vi "AlliGator Files Actions.vi"(0 "AlliGator Q Elements in":T5[](array[typedef]), 1 "VI in":refnum<vi>, 2 "Script in":bool, 5 "AlliGator IV DVR":refnum<data-value>, 7 "AlliGator Q Event in":T6=enum."GUI:Idle", 9 "Data":variant, 11 "error in (no error)":errorcluster, 12 "AlliGator Ctrl Refnums":T7) -> (3 "Script out":bool, 4 "AlliGator Q Elements out":T5[](array[typedef]), 6 "AlliGator IV DVR":refnum<data-value>, 10 "[Notebook Message]":T2[](array[typedef]) {"Message Style"."Text Alignment" items=["Left", "Right", "Center"]}, 15 "error out":errorcluster)   [LabVIEW 2021, in "AlliGator Action Engine.lvlib"]
doc: "Processes AlliGator files-related actions."
uses:
  AlliGator Action Engine.lvlib
  AlliGator Q Event.ctl
  AlliGator Ctrl Refnums.ctl
  AlliGator Other Ctrl Refnums.ctl
  AlliGator State Indicator.ctl
  AlliGator Phasor Plot Ctrl Refnums.ctl
  AlliGator Phasor Graph Ctrl Refnums.ctl
  Phasor/Phasor Calibration Type.ctl
  AlliGator Dataset Ctrl Refnums.ctl
  AlliGator Displayed Image.ctl
  AlliGator Registered Events Ctrl Refnums.ctl
  AlliGator Image Histogram Control Refnums.ctl
  Histograms/Linear Histogram Options.ctl
  Histograms/Histogram Bin Option.ctl
  Histograms/Histogram Bin Position.ctl
  AlliGator Decay Fit Map Control Refnums.ctl
  Fits/IRF(X)PSED/Decay Fit Parameters & Derived Quantities List.ctl
  AlliGator Q Element.ctl
  AlliGator Internal Variables v2.ctl
  <vilib>/vision/Image Controls.llb/IMAQ Image.ctl
  AlliGator Gate Image Set.ctl
  AlliGator FLI Dataset Type.ctl
  AlliGator Data Series Type.ctl
  AlliGator Dataset Channel.ctl
  AlliGator Gate Arithmetic.ctl
  Image/Named ROI Description.ctl
  AlliGator Decay Metadata v3.ctl
  AlliGator Decay Background Subtraction Info.ctl
  AlliGator Baseline Subtraction Method.ctl
  Graphs/XY Graph/XY Graph Plot Shift Parameters.ctl
  Graphs/XY Graph/XY Graph Plot Shift Method.ctl
  AlliGator Decay Extrapolation Parameters.ctl
  Phasor/Calibration Phasor (m, phi).ctl
  Phasor/Phasor Reference Series.ctl
  Phasor/Phasor Calibration Map v2.ctl
  Phasor/Phasor (g, s).ctl
  AlliGator Raw Phasor Plot Data v4.ctl
  Phasor/Phasor Standard Deviation Options.ctl
  AlliGator Phasor Multi-Harmonic Data.ctl
  Phasor/Phasor Harmonic Data.ctl
  AlliGator Decay Fit Options & Parameters v2.ctl
  Fits/IRF(X)PSED/Decay Fit Options v2.ctl
  Fits/Decay Convolution/Decay Model.ctl
  Fits/Residual Type.ctl
  Fits/IRF(X)PSED/Fit Weights Type.ctl
  Fits/Non-linear Fitting Method v2.ctl
  Fits/Fit Calculation Method.ctl
  Fits/Non-linear Fitting Algorithm.ctl
  AlliGator Decay Fit Parameter Constraints 2.ctl
  Fits/IRF(X)PSED/Decay Fit Parameters In List.ctl
  Fits/IRF(X)PSED/MLE Baseline Offset Type.ctl
  AlliGator Decay Preprocessing Parameters.ctl
  Notebook/Notebook Message Object.ctl
  Rich Text Box/Text Formatting.ctl
  Rich Text Box/Text Colors.ctl
  AlliGator Windows List.ctl
  Alligator Elements Order in Action Stack.ctl
  AlliGator Export Dataset Options.ctl
  AlliGator Variables List.ctl
  AlliGator Load Dataset Options.ctl
  AlliGator Single Image File Info.ctl
  AlliGator Image Type.ctl
  AlliGator Folder Selection.ctl
  AlliGator Select Folder Mode.ctl
  AlliGator Data Load & Process Options.ctl
  AlliGator Data Information.ctl
  AlliGator Gates to Skip.ctl
  AlliGator Define Gates to.ctl
  AlliGator Gates to Keep.ctl
  AlliGator Source Image Settings.ctl
  AlliGator Low Count Pixels Rejection Options.ctl
  AlliGator High Count Pixels Rejection Options.ctl
  AlliGator Image Smoothing Options.ctl
  Arrays/Kernel Type.ctl
  Arrays/Smoothing Algorithm.ctl
  AlliGator Image Binning Options.ctl
  AlliGator Decay Preprocessing Options.ctl
  AlliGator Background Subtraction Parameters.ctl
  AlliGator Settings List.ctl
  AlliGator Globals.vi
  AlliGator Add Action Array to Stack.vi
  Variant/Variant to Data/Variant to I32.vi
  Variant/Variant to Data/Variant to Path.vi
  AlliGator Add Single Action to Stack.vi
  Variant/Variant to Data/Variant to DBL.vi
  Variant/Variant to Data/Variant to Data.lvlib
  AlliGator GUI.lvlib
  Utilities/Utilities.lvlib
  GUI/GUI.lvlib
  AlliGator Files.lvlib
  AlliGator Source Image.lvlib
  AlliGator Scripts.lvlib
  Graphs/XY Graph/XY Graph Add-Ons.lvlib
  AlliGator Decay Preprocessing.lvlib
  Arrays/Arrays.lvlib
  AlliGator Settings.lvlib
  AlliGator Decay Analysis.lvlib
  AlliGator Globals, Variables & Constants.lvlib
  Rich Text Box/Rich Text Box.lvlib
  Image/Image.lvlib
  Phasor/Phasor.lvlib
  AlliGator Decay Fit Parameter Map.lvlib
  AlliGator Phasor Graph.lvlib
  AlliGator Phasor Plot.lvlib
  Fits/Fits.lvlib
  AlliGator Decay Fit.lvlib
  AlliGator Internal Variables.lvlib
  AlliGator Dual-Channel Datasets.lvlib
  Histograms/Histogram Window.lvlib
  Notebook/Notebook.lvlib
panel:
  in  "Displayed Image 2":T1=enum."Sum of All Gates" caption="Displayed Image"
  in  "Displayed Image":T1=enum."Sum of All Gates"
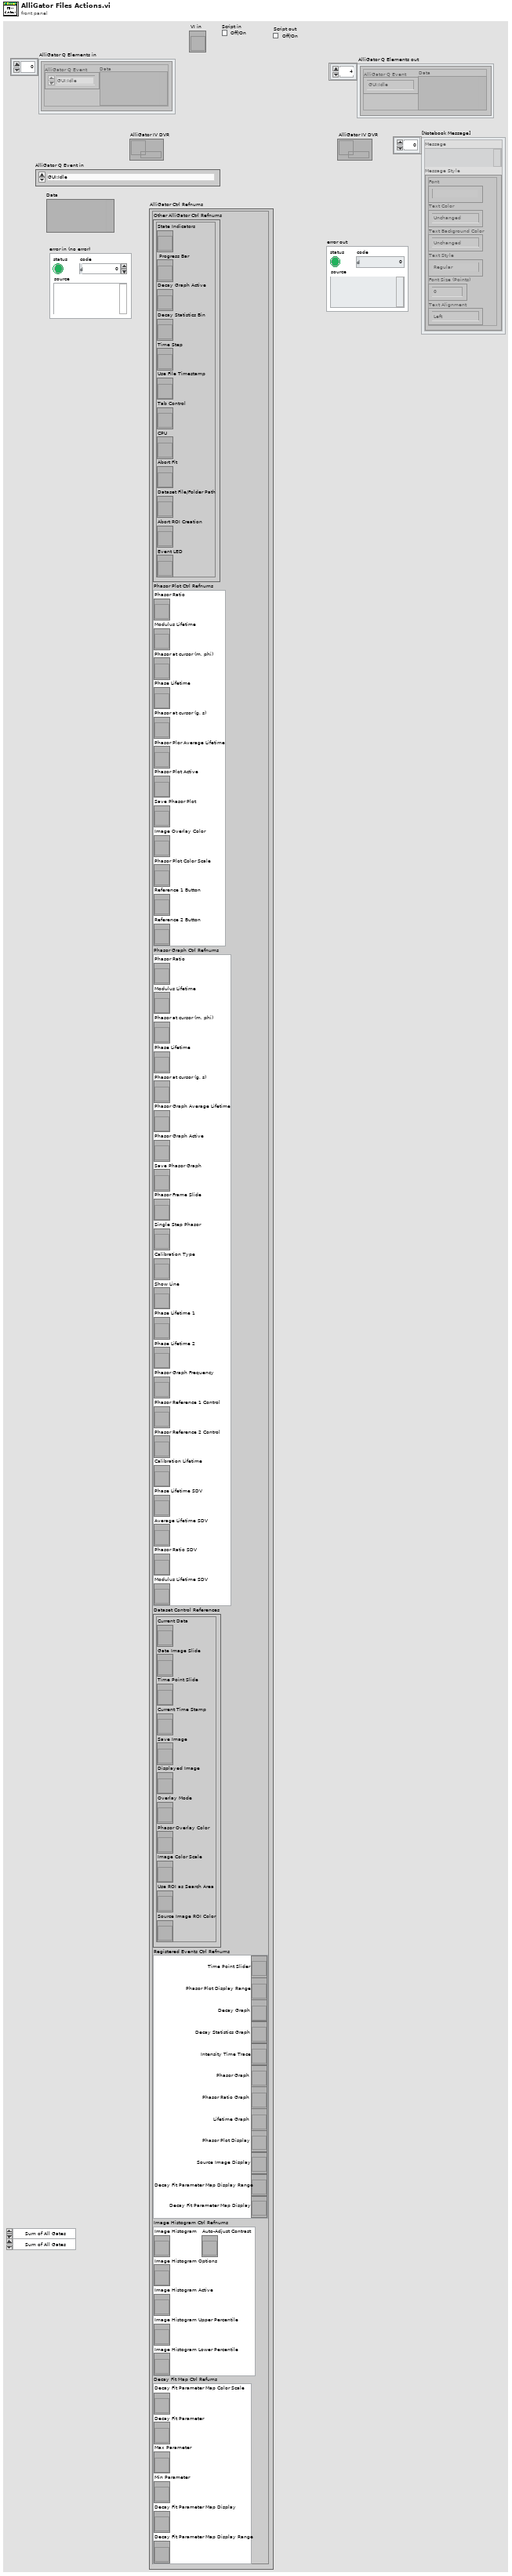
[diagram p1: front panel]
types:
  T1 = typedef "AlliGator Source Image.lvlib/AlliGator Displayed Image.ctl" = enum16{"Single Gate", "Sum of All Gates", "Max of All Gates", "Min of All Gates", "-", "White Ligth Image", "Mask Image"}
  T2 = typedef "Notebook.lvlib/Notebook Message Object.ctl" = cluster{"Message":string, "Message Style":T3}
  T3 = typedef "Rich Text Box.lvlib/Text Formatting.ctl" = cluster{"Font":string, "Text Color":T4, "Text Background Color":T4, "Text Style":enum16{"Regular", "Bold", "Italic", "Underline", "Strikeout"}, "Font Size (Points)":dbl, "Text Alignment":i32}
  T4 = typedef "Rich Text Box.lvlib/Text Colors.ctl" = enum16{"Unchanged", "Black", "Blue", "Brown", "Gray", "Green", "Orange", "Pink", "Red", "White"}
  T5 = typedef "AlliGator Action Engine.lvlib/AlliGator Q Element.ctl" = cluster{"AlliGator Q Event":T6, "Data":variant}
  T6 = typedef "AlliGator Action Engine.lvlib/AlliGator Q Event.ctl" = enum16{"---- Files ----", "Files:Set Batch Export Files To Save", "Files:Set Dataset Loading & Pre-processing Options", "Files:Check #Frames in Dataset", "Files:Increment Frame Index", "Files:Open Mask Image", "Files:Open White Light Image", "Files:Open Single Dataset", "Files:New Folder of Folders Selected", "Files:Load File (all Types)_Scriptable", "Files:Move Flattened Series to Folders Series", "Files:Select Folder", "Files:Load FLI Dataset", "Files:Load Swiss SPAD 1 Dataset", "Files:Load Swiss SPAD 2 Dataset", "Files:Load .sdt FLI Dataset", "Files:Load .ptu FLI Dataset", "Files:Load .bin FLI Dataset", "Files:Load Single Gate Image Folder", "Files:Load I/m/phi Dataset (deprecated)", "Files:Load Single Image", "Files:Subtract Background File", "Files:Export FLI Dataset", "Files:Load HDF5 FLI Dataset", "Files:Set Destination File Path", "Files:Save Mask Image", "Files:Batch Conversion", "Files:New Folder Selected", "Files:Close FLI Dataset", "Files:Close FLI Dataset Series", "Files:Close White Light Image", "Files:Close Mask Image", "---- FLI Dataset ----", "FLI Dataset:Channel Arithmetic", "FLI Dataset:Export Average Lifetime Map as ASCII", "FLI Dataset:Export User-Defined Quantity Map as ASCII", "FLI Dataset:Python Function FLI Dataset Event", "FLI Dataset:ROI Analysis", "FLI Dataset:Tilted Logistic Square Gated IRF Characteristics Map", "FLI Dataset:Logistic Square Gated IRF Characteristics Map", "FLI Dataset:Square Gated IRF Characteristics Map", "FLI Dataset:Multi-ROI Single-Pixel Phasor Analysis", "FLI Dataset:Multi-ROI Single-Pixel NLSF Analysis", "FLI Dataset:All ROIs IRF Extraction", "FLI Dataset:All ROIs Decay Fit Non-Interactive (Fast + Individual IRF)", "FLI Dataset:All ROIs Phasor Analysis", "FLI Dataset:All ROIs Decay Fit", "FLI Dataset:Fluorescence Decay Statistics", "FLI Dataset:Update Decay Statistics Graph", "FLI Dataset:Get Decay from ROI", "FLI Dataset:All ROIs Average Lifetimes", "---- FLI Dataset Series ----", "FLI Dataset Series:Sum All Datasets in Series", "FLI Dataset Series:Add Dataset to Accumulated Dataset", "FLI Dataset Series:Display Accumulated Dataset", "FLI Dataset Series:Clear Dataset Series Sum", "FLI Dataset Series:Time-Series Analysis (NLSF)", "FLI Dataset Series:Time-Series Analysis (Phasor)", "---- Image ----", "Image:Update Image Profile Plots", "Image:Image Histogram Cursor Move", "Image:Image Histogram", "Image:Image Contrast", "Image:Set Image Histogram Cursor Move Flag", "Image:Clear Image Overlay", "Image:Use ROI as Search Area", "Image:Set ROI Diameter", "Image:Save Image Data as TIFF", "Image:Save Displayed Image with Overlay", "Image:Save Image Overlay Only", "Image:Save Image as Hot Pixel Mask", "Image:Change Source Image Color Palette", "Image:Copy Image to Clipboard", "Image:Source Image ROI Selection", "Image:Delete All ROIs", "Image:Delete All Unselected ROIs", "Image:Delete ROI", "Image:Merge All ROIs", "Image:Store ROI", "Image:Source Image ROI Storage", "Image:Export ROI Description to Notebook", "Image:Save ROI", "Image:Load ROI", "Image:Paste ROI Definition", "Image:Clear ROI", "Image:Identify ROIs in Mask Image", "Image:Create Complementary ROI", "Image:Create Contour ROI", "Image:Create ROI(s) from Pixels with Peak above Min_Scriptable", "Image:Create ROI(s) from Pixels with Intensity above Min_Scriptable", "Image:Compute ROI Statistics", "Image:Delete ROI(s) based on ROI Characteristics", "Image:Create ROI Grid", "Image:ROI to Individual Pixel ROIs", "Image:Python Function Source Image Event", "Image:Show Phasor Calibration Map ROI Centers", "Image:Convert ROI to Mask Image", "Image:Mouse Move", "Image:Mouse Up", "Image:Set Source Image Mouse Move Flag", "Image:Add Scale Bar Overlay", "Image:Delete Existing ROIs Option", "---- Decay ----", "Decay:Clear IRF/Reference Plot", "Decay:Clear Local IRFs", "Decay:Add Decay to Graph", "Decay:Smoothen Plot", "Decay:Smoothen Plot Tail", "Decay:Average Selected Plots", "Decay:Extract IRF", "Decay:Optimal IRF Extraction", "Decay:Threshold IRF", "Decay:Fit to Model IRF", "Decay:Fit IRF to Square Gate", "Decay:Fit IRF to Logistic Square Gate", "Decay:Fit IRF to Tilted Logistic Square Gate", "Decay:Create Bounding Cursors Set", "Decay:Export Bounding Cursors Definition to Notebook", "Decay:Denoise Plot", "Decay:Compute Cumulative Function", "Decay:Use as Reference Decay", "Decay:Show Reference Decay/IRF", "Decay:Extrapolate Decay", "Decay:Create Head & Tail Bounding Cursors", "Decay:Store Cursor-defined Head & Tail Fractions", "Decay:Rebin Plot", "Decay:1-Normalize Decay", "Decay:[0-1]-Normalize Plot", "Decay:Straighten Decay", "Decay:Shift Decay", "Decay:Fold Decay", "Decay:Fit Decay", "Decay:Global Fit of Selected Decays", "Decay:Post Global Fit Script", "Decay:Add Global Fit Parameters to Graph", "Decay:Add Decay Parameter(s) to Plot (Graph)", "Decay:Export Decay to Phasor Graph", "Decay:Plot Decay Shifts", "Decay:Compute Average Lifetime", "Decay:Plot Convolution", "Decay:Graph Tip Strip Update", "---- Decay Statistics ----", "Decay Statistics:Tip Strip Update", "---- Intensity Time Trace ----", "Intensity Time Trace:Use File Timestamp", "Intensity Time Trace:Load Intensity Corrections File", "Intensity Time Trace:Clear Intensity Corrections File", "Intensity Time Trace:Tip Strip Update", "---- Phasor Plot ----", "Phasor Plot:Build Phasor Plot", "Phasor Plot:Change Phasor Plot Color Palette", "Phasor Plot:Adjust Phasor Plot Display Range", "Phasor Plot:Highlight Image ROI in Phasor Plot", "Phasor Plot:Save Phasor Plot Image with Overlay", "Phasor Plot:Export Complex Phasor Map", "Phasor Plot:Export Phasor Ratio Map", "Phasor Plot:Export Average Lifetime Map", "Phasor Plot:Compute Phase Lifetime Histogram", "Phasor Plot:Compute Phasor Ratio Histogram", "Phasor Plot:Compute Phase Lifetime vs Intensity Scatter Plot", "Phasor Plot:Weber 2-Component Decomposition", "Phasor Plot:Update Phasor Color Map Vertices", "Phasor Plot:Clear Phasor Overlay", "Phasor Plot:Use Segment Extremities as References", "Phasor Plot:Use UC/Segment Intersections as References", "Phasor Plot:Use UC/Principal Axis Intersections as References", "Phasor Plot:Use UC/Linear Fit Intersections as References", "Phasor Plot:Update Phasor Plot Reference", "Phasor Plot:Show Local Phasor Info in Phasor Plot", "Phasor Plot:Update Phasor Plot State", "Phasor Plot:Phasor Plot ROI Storage", "Phasor Plot:Phasor Plot ROI Selection", "Phasor Plot:Python Function Phasor Plot Event", "Phasor Plot:Overlay Phasor ROI, Ratio or Map in Source Image", "Phasor Plot:Compute Decay of Selected Phasors", "Phasor Plot:Phasor at Image Pixel", "Phasor Plot:Mouse Move", "Phasor Plot:Mouse Up", "Phasor Plot:Display Range Mouse Move", "Phasor Plot:Set Mouse Move Flag", "---- Phasor Graph ----", "Phasor Graph:Calibrated Phasor Map Series", "Phasor Graph:Whole Image Phasor Scatter Plot (Todo)", "Phasor Graph:Get Phasor Value", "Phasor Graph:Create New Phasor Plot Dialog", "Phasor Graph:Update Last Phasor Value", "Phasor Graph:Update Phasor (m, phi)", "Phasor Graph:Remove Single Phasor from Plot", "Phasor Graph:Add Single Phasor to Plot", "Phasor Graph:Remove Phasor Plot", "Phasor Graph:Remove Selected Phasor Plots", "Phasor Graph:Clear Phasor Data", "Phasor Graph:Clear Phasor Graph", "Phasor Graph:Cursor Move", "Phasor Graph:Draw Cursor Connecting Line", "Phasor Graph:Clear Cursor Connecting Line", "Phasor Graph:Find UC Intersection", "Phasor Graph:Use UC/Cursor-Defined Line Intersections", "Phasor Graph:Use Selected Plots Fitted Line/UC Intersections", "Phasor Graph:Use Selected Plots Principal Axis/UC Intersections", "Phasor Graph:Show Single Phasor", "Phasor Graph:Save Single Phasor Plot", "Phasor Graph:Save All Phasor Plots", "Phasor Graph:Load Phasor Plot(s)", "Phasor Graph:Phasor Multiplication", "Phasor Graph:Compute Average Phasor", "Phasor Graph:Compute Multiple Average Phasors (Selected Plots)", "Phasor Graph:Export Single Phasor Plot Phase Lifetimes", "Phasor Graph:Phase Lifetime Trajectory", "Phasor Graph:Phase Lifetime vs Intensity Scatter Plot (deprecated)", "Phasor Graph:Parameter 2 vs Parameter 1 Scatter Plot", "Phasor Graph:Use Cursor n Location", "Phasor Graph:Set Reference n to Current Phase Lifetime Value", "Phasor Graph:Set Reference n to Lifetime Value", "Phasor Graph:Set Cursor n Location", "Phasor Graph:Save Phasor Graph Image", "Phasor Graph:Update SEPL Plot", "Phasor Graph:Export Single Phasor Plot Data", "Phasor Graph:Export Selected Phasor Plots Data", "Phasor Graph:Python Function Phasor Graph Event", "Phasor Graph:Tip Strip Update", "---- Calibration ----", "Calibration:Set Calibration Type", "Calibration:Load/Save Phasor Calibration", "Calibration:Load/Save Phasor Calibration Series", "Calibration:Load/Save Phasor Calibration Map", "Calibration:Use as Calibration", "Calibration:Compute Optimal Calibration from Phasor References", "Calibration:Clear Phasor Calibration", "Calibration:Use as Calibration Series", "Calibration:Use as Calibration Map", "Calibration:Clear Calibration Series", "Calibration:Clear Calibration Map", "Calibration:Apply Phasor Calibration", "Calibration:Update Single Plot Calibration", "Calibration:Update Multiple Plots Calibration", "Calibration:Clear Single Plot Calibration", "Calibration:Clear All Plots Calibrations", "Calibration:Clear Plot(s) Calibration(s)?", "Calibration:Phasor Calibration Maps (# Gates Series)", "---- Phasor Ratio ----", "Phasor Ratio:Clear Reference n", "Phasor Ratio:Toggle Selected Plot(s)  Lock to Reference 1", "Phasor Ratio:Use as Reference n", "Phasor Ratio:Send Reference n to Notebook", "Phasor Ratio:Toggle Selected Plot(s)  Lock to Reference 2", "Phasor Ratio:Compute Phasor Ratio at Mouse Location", "Phasor Ratio:Compute Phasor Plot's Average Phasor Ratio", "Phasor Ratio:Compute Time-Series Phasor Ratios", "Phasor Ratio:Fit Line to Phasor Ratio Plot", "Phasor Ratio:Save References", "Phasor Ratio:Load References", "Phasor Ratio:Update Phasor Reference 1", "Phasor Ratio:Update Phasor Reference 2", "Phasor Ratio:Move Cursor n to Reference n", "Phasor Ratio:Use as Phasor Reference 1 Lifetime", "Phasor Ratio:Use as Phasor Reference 2 Lifetime", "Phasor Ratio:Export Phasor Ratio Map as ASCII", "Phasor Ratio:Tip Strip Update", "---- Lifetime & Other Parameters Graph ----", "Lifetime:Tip Strip Update", "---- Decay Fit Parameter Map ----", "Decay Fit Parameter Map:Export ROI NLSF Data as ASCII", "Decay Fit Parameter Map:Set Decay Fit  Parameter Map Selection", "Decay Fit Parameter Map:Build Decay Fit Parameter Map", "Decay Fit Parameter Map:Change Decay Fit Parameter Map Color Palette", "Decay Fit Parameter Map:Export Decay Fit Parameter Map Data as ASCII", "Decay Fit Parameter Map:Export All Decay Fit Parameter Maps Data as ASCII", "Decay Fit Parameter Map:Send Map Data to Lifetime Graph", "Decay Fit Parameter Map:Save Decay Fit Parameter Map Image", "Decay Fit Parameter Map:Save-Load IRFs & Fit Data", "Decay Fit Parameter Map:Update Local Decay Plots", "Decay Fit Parameter Map:Python Function Decay Fit Parameters Map Event", "Decay Fit Parameter Map:Overlay Decay Fit Parameter Map in Source Image", "Decay Fit Parameter Map:Plot Map Data vs Intensity", "Decay Fit Parameter Map:Mouse Up", "Decay Fit Parameter Map:Display Range Mouse Move", "---- Generic Graph ----", "Generic Graph:Generic XY Graph Event", "Generic Graph:Python Function XY Graph Event", "Generic Graph:New Plot", "Generic Graph:Save Plot", "Generic Graph:XY Plot Histogram", "Generic Graph:Set XY Graph Plot Name", "Generic Graph:Set Last Cursor Style", "Generic Graph:Tip Strip Update", "---- GUI ----", "GUI:Start Script", "GUI:Type of Displayed Image Changed", "GUI:Gate Image Slide Changed", "GUI:Show Busy Icon", "GUI:Show Busy Icon & Abort Button", "GUI:Hide Busy Icon", "GUI:Hide Busy Icon & Abort Button", "GUI:Abort", "GUI:End Script", "GUI:Start Timing", "GUI:End Timing", "GUI:Set State Indicator", "GUI:Send Parameters JSON Strings to Clipboard", "GUI:Set Gate Step", "GUI:Idle", "GUI:Initialization", "GUI:Quit", "GUI:Increment Dataset Index", "GUI:Set Dataset Index to -1", "GUI:Time Series Slider Moved", "GUI:Time Series Slider Changed", "GUI:Toggle Playback or Loop", "GUI:Playback Script", "GUI:Set Phasor Frequency", "GUI:Open Window", "DEBUG"}
  T7 = typedef "AlliGator GUI.lvlib/AlliGator Ctrl Refnums.ctl" = cluster{"Other AlliGator Ctrl Refnums":T8, "Phasor Plot Ctrl Refnums":T9, "Phasor Graph Ctrl Refnums":T10, "Dataset Control References":T11, "Registered Events Ctrl Refnums":T12, "Image Histogram Ctrl Refnums":T13, "Decay Fit Map Ctrl Refums":T14}
  T8 = typedef "AlliGator GUI.lvlib/AlliGator Other Ctrl Refnums.ctl" = cluster{"State Indicators":refnum<vi>, " Progress Bar":refnum<vi>, "Decay Graph Active":refnum<vi>, "Decay Statistics Bin":refnum<vi>, "Time Step":refnum<vi>, "Use File Timestamp":refnum<vi>, "Tab Control":refnum<vi>, "CPU":refnum<vi>, "Abort Fit":refnum<vi>, "Dataset File/Folder Path":refnum<vi>, "Abort ROI Creation":refnum<vi>, "Event LED":refnum<vi>}
  T9 = typedef "AlliGator GUI.lvlib/AlliGator Phasor Plot Ctrl Refnums.ctl" = cluster{"Phasor Ratio":refnum<vi>, "Modulus Lifetime":refnum<vi>, "Phasor at cursor (m, phi)":refnum<vi>, "Phase Lifetime":refnum<vi>, "Phasor at cursor (g, s)":refnum<vi>, "Phasor Plor Average Lifetime":refnum<vi>, "Phasor Plot Active":refnum<vi>, "Save Phasor Plot":refnum<vi>, "Image Overlay Color":refnum<vi>, "Phasor Plot Color Scale":refnum<vi>, "Reference 1 Button":refnum<vi>, "Reference 2 Button":refnum<vi>}
  T10 = typedef "AlliGator GUI.lvlib/AlliGator Phasor Graph Ctrl Refnums.ctl" = cluster{"Phasor Ratio":refnum<vi>, "Modulus Lifetime":refnum<vi>, "Phasor at cursor (m, phi)":refnum<vi>, "Phase Lifetime":refnum<vi>, "Phasor at cursor (g, s)":refnum<vi>, "Phasor Graph Average Lifetime":refnum<vi>, "Phasor Graph Active":refnum<vi>, "Save Phasor Graph":refnum<vi>, "Phasor Frame Slide":refnum<vi>, "Single Step Phasor":refnum<vi>, "Calibration Type":refnum<vi>, "Show Line":refnum<vi>, "Phase Lifetime 1":refnum<vi>, "Phase Lifetime 2":refnum<vi>, "Phasor Graph Frequency":refnum<vi>, "Phasor Reference 1 Control":refnum<vi>, "Phasor Reference 2 Control":refnum<vi>, "Calibration Lifetime":refnum<vi>, "Phase Lifetime SDV":refnum<vi>, "Average Lifetime SDV":refnum<vi>, "Phasor Ratio SDV":refnum<vi>, "Modulus Lifetime SDV":refnum<vi>}
  T11 = typedef "AlliGator GUI.lvlib/AlliGator Dataset Ctrl Refnums.ctl" = cluster{"Current Data":refnum<vi>, "Gate Image Slide":refnum<vi>, "Time Point Slide":refnum<vi>, "Current Time Stamp":refnum<vi>, "Save Image":refnum<vi>, "Displayed Image":refnum<vi>, "Overlay Mode":refnum<vi>, "Phasor Overlay Color":refnum<vi>, "Image Color Scale":refnum<vi>, "Use ROI as Search Area":refnum<vi>, "Source Image ROI Color":refnum<vi>}
  T12 = typedef "AlliGator GUI.lvlib/AlliGator Registered Events Ctrl Refnums.ctl" = cluster{"Time Point Slider":refnum<vi>, "Phasor Plot Display Range":refnum<vi>, "Decay Graph":refnum<vi>, "Decay Statistics Graph":refnum<vi>, "Intensity Time Trace":refnum<vi>, "Phasor Graph":refnum<vi>, "Phasor Ratio Graph":refnum<vi>, "Lifetime Graph":refnum<vi>, "Phasor Plot Display":refnum<vi>, "Source Image Display":refnum<vi>, "Decay Fit Parameter Map Display Range":refnum<vi>, "Decay Fit Parameter Map Display":refnum<vi>}
  T13 = typedef "AlliGator GUI.lvlib/AlliGator Image Histogram Control Refnums.ctl" = cluster{"Image Histogram":refnum<vi>, "Image Histogram Options":refnum<vi>, "Image Histogram Active":refnum<vi>, "Image Histogram Upper Percentile":refnum<vi>, "Image Histogram Lower Percentile":refnum<vi>, "Auto-Adjust Contrast":refnum<vi>}
  T14 = typedef "AlliGator Decay Fit Parameter Map.lvlib/AlliGator Decay Fit Map Control Refnums.ctl" = cluster{"Decay Fit Parameter Map Color Scale":refnum<vi>, "Decay Fit Parameter":refnum<vi>, "Max Parameter":refnum<vi>, "Min Parameter":refnum<vi>, "Decay Fit Parameter Map Display":refnum<vi>, "Decay Fit Parameter Map Display Range":refnum<vi>}
  T15 = typedef "AlliGator GUI.lvlib/AlliGator Windows List.ctl" = enum16{"AlliGator Window", "Settings Window", "Notebook Window", "Dataset Information Window", "Source Image ROI Manager Window", "Phasor Plot ROI Manager Window", "Phasor Harmonic Manager Window", "Histogram Window", "Image Profile Window", "Local Decay Window", "About Window", "Batch Conversion Window", "Shot Noise Influence on Average Lifetime", "Fit Method Benchmark", "AlliGator Alias Definition"}
  T16 = typedef "AlliGator Action Engine.lvlib/Alligator Elements Order in Action Stack.ctl" = enum16{"Enqueue 2 AFTER 1", "Enqueue 2 BEFORE 1"}
  T17 = typedef "AlliGator Files.lvlib/AlliGator Export Dataset Options.ctl" = cluster{"Destination File Type":string, "Dialog?":bool}
  T18 = typedef "AlliGator Files.lvlib/AlliGator Load Dataset Options.ctl" = cluster{"FLI Dataset Type":T19, "No Dialog?":bool, "File Path":path}
  T19 = typedef "AlliGator Files.lvlib/AlliGator FLI Dataset Type.ctl" = enum16{"HDF5 FLI Dataset", "Gate Image Folder", ".sdt FLI Dataset (Becker & Hickl)", ".ptu FLI Dataset (PicoQuant)", "SS1 FLI Dataset", "SS2 FLI Dataset", "I/m/phi Dataset", ".bin FLI Dataset (PicoQuant Binned)", ".bin FLI Dataset (Piccolo Binned)"}
  T20 = typedef "AlliGator Files.lvlib/AlliGator Single Image File Info.ctl" = cluster{"Image Type":T21, "Image Path":path}
  T21 = typedef "AlliGator Source Image.lvlib/AlliGator Image Type.ctl" = enum16{"White Light Image", "Mask Image"}
  T22 = typedef "AlliGator Files.lvlib/AlliGator Folder Selection.ctl" = cluster{"Folder Selection Mode":T23, "Folder Path":path}
  T23 = typedef "AlliGator Files.lvlib/AlliGator Select Folder Mode.ctl" = enum16{"Select Gate Folder", "Select Folder of Gate Folders", "Select Folder of SwissSPAD 2 Datasets", "Select Folder of .sdt FLI Datasets (Becker & Hickl)", "Select Folder of .ptu FLI Datasets (PicoQuant)", "Select Folder of .bin FLI Datasets (PicoQuant Binned)", "Select Folder of .bin FLI Datasets (Piccolo Binned)", "Select Folder of HDF5 FLI Datasets"}
  T24 = typedef "AlliGator Scripts.lvlib/AlliGator Data Load & Process Options.ctl" = cluster{"Data Information":T25, "Source Image Settings":T30, "Decay Preprocessing Options & Parameters":T37, "Clear Phasor Graph":bool}
  T25 = typedef "AlliGator Scripts.lvlib/AlliGator Data Information.ctl" = cluster{"Gates to Skip":T26, "# Gates":u32, "Gate Step":u32, "Gate Duration":dbl[unit], "Gate Separation":dbl[unit], "Pile-up Correction":bool, "Pixel Well Capacity":u32, "Define Gates to":T27, "Gates to Keep":T28, "Laser Period":dbl[unit], "SYNC Period":dbl[unit], "Channel Name":u16, "Channel Arithmetic":T29, "Background File Subtraction":bool, "Background Scaling Factor":dbl, "Background File":path, "Background Pile-up Correction":bool, "Background Pixel Well Capacity":u32, "Dataset Scaling Factor":dbl}
  T26 = typedef "AlliGator Decay Analysis.lvlib/AlliGator Gates to Skip.ctl" = cluster{"Start":u32, "End":u32}
  T27 = typedef "AlliGator Settings.lvlib/AlliGator Define Gates to.ctl" = enum32{"Skip", "Keep"}
  T28 = typedef "AlliGator Settings.lvlib/AlliGator Gates to Keep.ctl" = cluster{"First":u32, "Last":u32}
  T29 = typedef "AlliGator Settings.lvlib/AlliGator Gate Arithmetic.ctl" = enum16{"None", "INT-G2", "G2/INT*<INT>", "(1 - G2/INT)*<INT>"}
  T30 = typedef "AlliGator Scripts.lvlib/AlliGator Source Image Settings.ctl" = cluster{"Low Count Pixels Rejection Options":T31, "High Count Pixels Rejection Options":T32, "Peak Threshold":dbl, "Intensity Threshold":dbl, "Image Smoothing Options":T33, "Image Binning Options":T36}
  T31 = typedef "AlliGator Settings.lvlib/AlliGator Low Count Pixels Rejection Options.ctl" = cluster{"Background Low Threshold Factor":dbl, "Fixed Low Background Threshold":dbl, "Reject Low Count Pixels":bool, "Low Percentile":dbl}
  T32 = typedef "AlliGator Settings.lvlib/AlliGator High Count Pixels Rejection Options.ctl" = cluster{"Background High Threshold Factor":dbl, "Fixed High Background Threshold":dbl, "Reject High Count Pixels":bool, "High Percentile":dbl}
  T33 = typedef "AlliGator Settings.lvlib/AlliGator Image Smoothing Options.ctl" = cluster{"Use Image Smoothing":bool, "Kernel Type":T34, "Bin":i32, "Algorithm":T35}
  T34 = typedef "Arrays.lvlib/Kernel Type.ctl" = enum16{"Uniform", "Bilinear", "Gaussian"}
  T35 = typedef "Arrays.lvlib/Smoothing Algorithm.ctl" = enum16{"Rapid", "Thorough"}
  T36 = typedef "AlliGator Source Image.lvlib/AlliGator Image Binning Options.ctl" = cluster{"Use Image Binning":bool, "X Bin":i32, "Y Bin":i32}
  T37 = typedef "AlliGator Decay Analysis.lvlib/AlliGator Decay Preprocessing.lvlib/AlliGator Decay Preprocessing Options.ctl" = cluster{"Background Subtraction Parameters":T38, "Decay Preprocessing Parameters":T40, "Preprocessing Steps Order":string[]}
  T38 = typedef "AlliGator Decay Analysis.lvlib/AlliGator Decay Preprocessing.lvlib/AlliGator Background Subtraction Parameters.ctl" = cluster{"Background Definition Range":cluster{"Min Gate":dbl[unit], "Max Gate":dbl[unit]}, "Baseline Subtraction Method":T39, "Background Subtraction?":bool, "Background File":path, "Background Constant":dbl, "Background Scaling Factor":dbl, "Background Pile-up Correction":bool, "Background Pixel Well Capacity":u32}
  T39 = typedef "AlliGator Decay Analysis.lvlib/AlliGator Decay Preprocessing.lvlib/AlliGator Baseline Subtraction Method.ctl" = enum16{"Mean", "Min", "Square Gated Single-Exponential", "File", "Constant"}
  T40 = typedef "AlliGator Decay Analysis.lvlib/AlliGator Decay Preprocessing.lvlib/AlliGator Decay Preprocessing Parameters.ctl" = cluster{"Background Subtraction":bool, "Straighten Decay":bool, "Reverse Gates":bool, "1-Normalized Decay":bool, "Smoothen Decay":bool, "Smoothing Parameter":dbl, "Shift Decay":bool, "Decay Shift Parameters":T41, "Extrapolate Decay":bool, "Additional Points":u32, "Head Fraction":dbl, "Pixel-Normalize Decay":bool, "Use Periodicity":bool, "Use Cursors":bool, "Tail Fraction":dbl, "Use Decay Pre-Processing":bool, "Fold Decay":bool, "# Folds":u32, "[0-1]-Normalized Decay":bool}
  T41 = typedef "XY Graph Add-Ons.lvlib/XY Graph Plot Shift Parameters.ctl" = cluster{"Type":T42, "Shift":dbl[unit], "Threshold":dbl, "Rotate":bool}
  T42 = typedef "XY Graph Add-Ons.lvlib/XY Graph Plot Shift Method.ctl" = enum16{"Default", "CFD", "Threshold", "Cross-Correlation"}
  T43 = typedef "AlliGator Globals, Variables & Constants.lvlib/AlliGator Variables List.ctl" = enum16{"---- GUI ----", "Initialization Status", "State Indicators Refnum", "Original AlliGator Menu Items", "Current Action Loop State", "Script in progress", "Playback", "Loop Playback", "Search ROI Used", "Search ROI", "Decay Graph Max Legend Size", "Intensity Graph Max Legend Size", "Decay Statistics Graph Max Legend Size", "Phasor Graph Max Legend Size", "Phasor Ratio Graph Max Legend Size", "Lifetime Graph Max Legend Size", "---- Files ----", "Export Dataset Frames as Individual Files", "Show Batch Export Help Balloons", "Frames in Dataset", "ptu File Frame Start Indices", "Current Frame in Dataset", "Current Frame Timestamp", "------ Python Plugins ------", "Python Plugins Information", "Python Session", "Valid Python Session?", "---- Source Image ----", "Dataset Loaded", "Dataset Metadata", "Dataset Channel", "Dataset Data Description", "Background Dataset Metadata", "Background Dataset Channel", "Background Dataset Data Description", "Background File Subtraction", "Background File Path", "Background File Pile-up Correction", "Background File Pixel Well Capacity", "Background File Scaling Factor", "Source Image ROIs", "Current Source Image ROI", "Source Image ROI Event Refnum", "X_Source Image Display Range", "X_Source Image Palette Information", "Source Image Palette List", "Source Image Scale", "Current Dataset Load Settings", "Source Image:ROI Overlay Color", "---- Image Profile Window ----", "Image Profile:Overlay ROI in Source Image", "Image Profile Window Event Refnum", "Image Profile:IntensityType", "Image Profile:Intensity Average Type", "Image Profile:Intensity-weighted SDV", "Image Profile:Box Profile Type", "Image Profile Window Open", "Image Profile:Plotted Fit Parameter", "X_Type of Displayed Image", "X_Time Gate Slider", "Dataset Path", "Source Image Overlay to Erase", "Is Displayed Image Accumulated", "White Light Image Modified", "Mask Image Modified", "Macrotime Gate Separation", "------ Phasor Graph -------", "Phasor Graph:Show Line", "---- Phasor Plot ---", "Phasor Plot Parameters Changed", "FLI Dataset Modified since last Phasor Plot Calculation", "Phasor Harmonics Data", "Selected Phasor Harmonics", "Phasor Harmonic Manager Event Refnum", "Phasor Plot ROIs", "Current Phasor Plot ROI", "Phasor Plot ROI Event Refnum", "Phasor Plot Image Reference Points", "Phasor Plot Computed", "Phasor Plot Palette Information", "Phasor Plot Palette List", "Phasor Ratio Palette Information", "Phasor Ratio Palette List", "Phasor Image Scale", "Phasor Plot Image Overlay to Erase", "Phasor Plot Image Elements to Update", "Current Phasor Plot Calculation Parameters", "Current Phasor Calibration Options", "Reset Cumulated Phasor Plot", "Phasor Ratio Reference 1", "Phasor Ratio Lifetime Reference 1", "Phasor Ratio Reference 1 Frequency", "Phasor Ratio Reference 2", "Phasor Ratio Lifetime Reference 2", "Phasor Ratio Reference 2 Frequency", "---- Decay Analysis ----", "Number of Selected Decays to Fit", "LS Fit Results", "LAR Fit Results", "BS Fit Results", "Last Decay Max - Min", "Best Fit Parameters", "Best Fit Parameter Names", "Actual Size X", "Actual Size Y", "Binning X", "Binning Y", "Actual # Gates", "Dataset Number", "Gates to...", "Gates Skipped", "Gates to keep", "Gate Step", "Gate Separation", "Reversed Gates", "Pile-up Correction", "Pixel Well Capacity", "Background Subtracted", "Background Subtraction Method", "Background Definition Range", "Background File (deprecated)", "Number of Dataset Accumulated", "Array of Accumulated Dataset Paths", "Do Averaged Datasets", "Destination File Path", "Process Plot Target", "Use 1/D as Phasor Frequency", "---- Decay Fit Parameter Map -----", "Decay Fit Parameter Map Palette Information", "Decay Fit Parameter Map Palette List", "Local Decay Graph Window Event Refnum", "------- Local Decay Window ---------", "Use normalized IRF for convolution", "----- Miscellaneous ----", "Skippable Dialog Windows Status"}
  T44 = typedef "AlliGator Settings.lvlib/AlliGator Settings List.ctl" = enum16{"GUI:Visible Settings Tab", "GUI:Last Run Version", "Source Image:Use Image Histogram for Contrast", "Source Image:Low Count Pixels Rejection Options", "Source Image:High Count Pixels Rejection Options", "Source Image:Use Image Brightness", "Source Image:Blend Overlay with Image Background", "Source Image:Use Fixed ROI Diameter", "Source Image:ROI Diameter", "Source Image:ROI Center Color", "Source Image:Peak Threshold", "Source Image:Intensity Threshold", "Source Image:Image Binning Options", "Source Image:Image Smoothing Options", "Source Image:Image Histogram Active", "Source Image:Invert Binary Mask", "Source Image:Hot Pixel Removal", "Source Image:Overlay Analyzed ROI Center", "Source Image:Auto-Adjust Contrast", "Source Image:Histogram Lower Percentile", "Source Image:Histogram Upper Percentile", "Source Image:Save Source Image", "Source Image:Scale Bar Options", "Source Image:Image Resolution (Pixel Size)", "Source Image:Flatfield Correction", "Data Information:Gate Width", "Data Information:Nanotime Gate Separation", "Data Information:Macrotime Gate Separation", "Data Information:Gate Step", "Data Information:# Gates", "Data Information:Gate Image Exposure", "Data Information:Gate Image Integration", "Data Information:Gates to Skip", "Data Information:Gates to Keep", "Data Information:Define Gates to", "Data Information:Channel Name", "Data Information:Available Channel Names", "Data Information:Channel Arithmetic", "Data Information:Background File Subtraction", "Data Information:Background File", "Data Information:Background Scaling Factor", "Data Information:Background Pile-up Correction", "Data Information:Background Pixel Well Capacity", "Data Information:Laser Period", "Data Information:SYNC Period", "Data Information:Pile-up Correction", "Data Information:Pixel Well Capacity", "Data Information:Dataset Scaling Factor", "Fluorescence Decay_Decay Pre-Processing:Reverse Gates", "Fluorescence Decay_Decay Pre-Processing:Verbose Decay Pre-Processing", "Fluorescence Decay_Decay Pre-Processing:Use Decay Pre-Processing", "Fluorescence Decay_Decay Pre-Processing:Background Subtraction", "Fluorescence Decay_Decay Pre-Processing:Background Definition Range", "Fluorescence Decay_Decay Pre-Processing:Baseline Subtraction Method", "Fluorescence Decay_Decay Pre-Processing:Operations Order", "Fluorescence Decay_Decay Pre-Processing:Smoothing Parameter", "Fluorescence Decay_Decay Pre-Processing:Shift Decay", "Fluorescence Decay_Decay Pre-Processing:Decay Shift Parameters", "Fluorescence Decay_Decay Pre-Processing:Fold Decay", "Fluorescence Decay_Decay Pre-Processing:# Folds", "Fluorescence Decay_Decay Pre-Processing:1-Normalize Decay", "Fluorescence Decay_Decay Pre-Processing:[0-1]-Normalize Decay", "Fluorescence Decay_Decay Pre-Processing:Smoothen Decay", "Fluorescence Decay_Decay Pre-Processing:Extrapolate Decay", "Fluorescence Decay_Decay Pre-Processing:Use Periodicity", "Fluorescence Decay_Decay Pre-Processing:Use Cursors", "Fluorescence Decay_Decay Pre-Processing:Tail Fraction", "Fluorescence Decay_Decay Pre-Processing:Head Fraction", "Fluorescence Decay_Decay Pre-Processing:Additional Points", "Fluorescence Decay_Decay Pre-Processing:Straighten Decay", "Fluorescence Decay_Decay Pre-Processing:Constant Background", "Fluorescence Decay_Decay Pre-Processing:Pixel-Normalize Decay", "Fluorescence Decay_Advanced Analysis:Extract IRF instead of Decay", "Fluorescence Decay_Advanced Analysis:IRF Extraction Options", "Fluorescence Decay_Advanced Analysis:IRF Optimization Options", "Fluorescence Decay_Advanced Analysis:Square Pulse Options", "Fluorescence Decay_Advanced Analysis:IRF Order", "Fluorescence Decay_Advanced Analysis:IRF Time Constants", "Fluorescence Decay_Advanced Analysis:Wavelet Analysis Options", "Fluorescence Decay_Advanced Analysis:Average Lifetime Options", "Fluorescence Decay_Fit Options:Fit Options", "Fluorescence Decay_Fit Options:Use Legacy Fitting Approach", "Fluorescence Decay_Fit Options:Use Data Information Laser Period", "Fluorescence Decay_Fit Parameters:Displayed Fit Parameters", "Fluorescence Decay_Fit Parameters:Fit Parameter Constraints", "Fluorescence Decay_Fit Parameters:Export Tabulated Results", "Fluorescence Decay_Fit Parameters:MLE Baseline Offset Type", "Fluorescence Decay_Fit Parameters:MLE Baseline Offset", "Fluorescence Decay_Fit Parameters:Guess Parameter Names", "Fluorescence Decay_Fit Parameters:Guess Parameter Values", "Fluorescence Decay_Fit Parameters:Guess Parameters Options", "Fluorescence Decay_Styles:Show Last Decay Only", "Fluorescence Decay_Styles:Decay Graph Color Array", "Fluorescence Decay:Decay Graph Active", "Fluorescence Decay Statistics:Min Peak Value", "Fluorescence Decay Statistics:Reject Low Decay Peak Pixels", "Fluorescence Decay Statistics:Reject High Decay Peak Pixels", "Fluorescence Decay Statistics:Max Peak Value", "Time Traces:Use File Timestamp", "Time Traces:Time Step", "Time Traces:Use Intensity Correction File", "Time Traces:Intensity Correction File", "Phasor Plot:Phasor Plot Smoothing Options", "Phasor Plot:Phasor Plot Size", "Phasor Plot:Phasor Plot Graphics Options", "Phasor Plot:Cumulative Phasor Plot", "Phasor Plot:Use Phasor Brightness", "Phasor Plot:Blend Overlay with Phasor Background", "Phasor Plot:Save Phasor Plot", "Phasor Plot:Show References", "Phasor Plot:Phasor Ratio Decay Range", "Phasor Plot:Exponential Fading", "Phasor Plot:Phasor Ratio Reference Colors", "Phasor Plot:Reference Radius", "Phasor Plot:Show Color Map Vertices", "Phasor Plot:Phasor Plot Active", "Phasor Plot:Phasor Ratio Color Map Type", "Phasor Plot:Phasor Ratio Color Map", "Phasor Plot:Phasor Ratio Display Range", "Phasor Plot:Selected Image ROI(s)", "Phasor Plot:All Image ROIs", "Phasor Plot:Selected Phasor Plot ROI(s)", "Phasor Plot:All Phasor Plot ROIs", "Phasor Plot:Phasor Ratio Color-Coded Quantity", "Phasor Plot:Store Phasor Harmonics", "Phasor Plot:Draw Reference Segment", "Phasor Plot:User-Defined Quantity", "Phasor Graph:Phasor Frequency", "Phasor Graph:Phasor Ratio Type", "Phasor Graph:Pixel-level Phasor Computation", "Phasor Graph:Save Phasor Graph", "Phasor Graph:Phasor Graph Active", "Phasor Graph:Phasor SDV Options", "Phasor Calibration:Use Backup Calibration if needed", "Phasor Graph:Define Shortest Lifetime as", "Phasor Calibration:Backup Calibration Type", "Phasor Calibration:Calibration Type", "Phasor Calibration:Calibration Lifetime", "Phasor Calibration:Calibration Map Algorithm", "Single-Exponential Phasor Locus (SEPL):Gate Parameters", "Single-Exponential Phasor Locus (SEPL):User-defined Gate", "Single-Exponential Phasor Locus (SEPL):User-defined IRF", "Single-Exponential Phasor Locus (SEPL):Phasor Parameters", "Single-Exponential Phasor Locus (SEPL):Decay & IRF Parameters", "Single-Exponential Phasor Locus (SEPL):Display Parameters", "Lifetime Analysis:Decay Analysis Parameters", "Lifetime Analysis:Lifetime Map Active", "Plugins:Python Settings", "Miscellaneous:Verbose Mode", "Miscellaneous:Beep after Script", "Miscellaneous:Saved Image File Format", "Miscellaneous:Exported Gate Image Settings", "Miscellaneous:Include Loading in Timing", "Miscellaneous:Verbose Settings Mode", "Miscellaneous:Histogram Options", "Miscellaneous:Beep on Error", "Miscellaneous:# Logical Processors Used", "Miscellaneous:ROI Description Max Characters", "Miscellaneous:Verbose Error Mode", "Miscellaneous:Transparent Mask Color"}
  T45 = typedef "AlliGator Internal Variables.lvlib/AlliGator Internal Variables v2.ctl" = cluster{"Displayed Image":T46, "White Light Image":T46, "Mask Image":T46, "ROI Mask Image":T46, "Current Dataset Images 1":T47, "Background Dataset Images 1":T47, "Current Dataset Images 2":T47, "Background Dataset Images 2":T47, "Current Dataset Arithmetic Images":T47, "Accumulated Dataset Images 1":T47, "Accumulated Dataset Images 2":T47, "Accumulated Dataset Arithmetic Images":T47, "Phasor Plot Image":T46, "Decay Fit Parameter Map Image":T46, "Single Data Point Path":path, "White Light Image Path":path, "Mask Image Path":path, "Time-Series Folder":path, "[Time-Series Paths]":path[], "Current Dataset":i32, "Single Dataset Type":T19, "Current Folder":string, "AlliGator Data Series Type":T48, "# Datasets":i32, "Dual-Channel Dataset":bool, "Selected Channel Name":string, "Dataset Channel":T49, "Channel Arithmetic":T29, "Dual-Channel Background Dataset":bool, "Background Channel":T49, "Dual-Channel Accumulated Dataset":bool, "Start Time":dbl, "[Time-Series Timestamps]":dbl[], "[Intensity Corrections]":dbl[], "Time Series Script":bool, "Type of Displayed Image":T1, "Gate Image Slide":u16, "# Gates":i32, "ROIs":T50[], "ROI Decay":cluster{"t Array":dbl[], "I Array":dbl[]}, "Valid Decay":bool, "Decay  Metadata":T52, "Reference Decay Plot Name":string, "Reference Decay":cluster{"t Array":dbl[], "I Array":dbl[]}, "Decay Shift Plot":cluster{"Time Stamps":dbl[], "Decay Shifts":dbl[]}, "[Decays Max Values]":sgl[], "[Decays Min Values]":sgl[], "Calibration Phasor":T55, "Calibration Phasor Series":T56, "Phasor Calibration Map":T57, "Calibration Map MD5 Digest":string, "Last Raw Phasor":T58, "Last Calibrated Phasor":T58, "Last Calibrated Phasor SDV":T58, "Phasor Graph:Phasor Plot":cluster{"g Array":dbl[], "s Array":dbl[]}, "Phasor Graph:Phasor SDV Plot":cluster{"g Array":dbl[], "s Array":dbl[]}, "[Phasor Graph:Raw Phasor Plots]":T59[], "Phasor Plot locked to Ref 1":i32, "[Phasor Plot(s) locked to Ref 1]":i32[], "[Phasor Plot(s) locked to Ref 2]":i32[], "[Pixel Phasors]":T58[], "[[Sum Image]]":dbl[][], "[[CSG Phasors]]":csg[][], "[[Valid Pixel?]]":bool[][], "I/m/phi Dataset":cluster{"I/m/phi Dataset?":bool, "Base Frequency":dbl[unit], "Harmonic Orders":u8[]}, "Multi Phasor Plot Data":T61, "Decay Fit Options & Parameters":T63, "Fit Options: Decay Preprocessing Parameters":T40, "Fit Options: Reference Decay":cluster{"t Array":dbl[], "I Array":dbl[]}, "Is Full Image Parameters Map":bool, "Is Single-Pixels Parameters Map":bool, "NLSF Parameters Map X Resolution":i32, "NLSF Parameters Map Y Resolution":i32, "[Single Decay Fit Parameters]":dbl[], "Fit Model":T65, "[[Multiple Decays Fit Parameters]]":dbl[][], "[[Multiple Decays Fit Parameter SDVs]]":dbl[][], "[[IRFs]]":dbl[][], "IRF Array Time Axis":dbl[], "Decay Array Time Axis":dbl[], "[Decay Fit Parameter Names]":T74[], "[[Phasor Ratios]]":dbl[][], "[[Average Lifetimes]]":dbl[][], "Amplitude Weighted Average Lifetime":bool, "[Decay Sum]":dbl[], "[[User-defined Quantities]]":dbl[][], "User-defined Quantity":string}
  T46 = typedef "IMAQ Image.ctl" = refnum<image>
  T47 = typedef "AlliGator Files.lvlib/AlliGator Gate Image Set.ctl" = cluster{"SGL Image Max":T46, "SGL Image Sum":T46, "SGL Gate Images":T46[], "SGL Image Min":T46}
  T48 = typedef "AlliGator Files.lvlib/AlliGator Data Series Type.ctl" = enum16{"Not a Supported Series", "Gate Images Folder Series", "SwissSPAD 2 Dataset Series", "B&H FLI Dataset Series", "PicoQuant PTU FLI Dataset Series", "PicoQuant BIN FLI Dataset Series", "Piccolo hist BIN FLI Dataset Series", "HDF5 FLI Dataset Series"}
  T49 = typedef "AlliGator Dual-Channel Datasets.lvlib/AlliGator Dataset Channel.ctl" = enum16{"G2", "INT"}
  T50 = typedef "Image.lvlib/Named ROI Description.ctl" = cluster{"ROI Descriptor":T51, "ROI Name":string, "Overlay Color":u32}
  T51 = typedef "ROI Descriptor" = cluster{"Global Rectangle":i32[], "Contours":cluster{"ID":enum32{"External", "Internal"}, "Type":u32, "Coordinates":i32[]}[]}
  T52 = typedef "AlliGator Phasor Graph.lvlib/AlliGator Decay Metadata v3.ctl" = cluster{"ROI Descriptor":T51, "ROI Center":cluster{"X":i32, "Y":i32}, "Decay Background Subtraction Info":T53, "Decay Reverted":bool, "Decay Smoothened":bool, "Decay Straightened":bool, "Fitted Tau (Decay Straightening)":dbl, "Decay Shift Parameters":T41, "Decay Shifted":bool, "Decay Extrapolated":bool, "Decay Extrapolation Parameters":T54, "Decay Normalized":bool, "Fold Decay":bool, "# Folds":u32}
  T53 = typedef "AlliGator Decay Analysis.lvlib/AlliGator Decay Preprocessing.lvlib/AlliGator Decay Background Subtraction Info.ctl" = cluster{"Laser Period":dbl[unit], "Gate Duration":dbl[unit], "Baseline Subtraction Method":T39, "Background Definition Range":cluster{"Min Gate":dbl[unit], "Max Gate":dbl[unit]}, "Total Intensity w/o Bkgd Subtraction":dbl, "Bkgd-subtracted Intensity (exp)":dbl, "# Data Points":i32, "Background/Gate":dbl, "Fitted Lifetime":dbl[unit], "Bkgd-subtracted Intensity (theo)":dbl}
  T54 = typedef "AlliGator Decay Analysis.lvlib/AlliGator Decay Preprocessing.lvlib/AlliGator Decay Extrapolation Parameters.ctl" = cluster{"Additional Points":u32, "Head Fraction":dbl, "Fitted Tau":dbl, "Use Periodicity":bool, "Use Cursors":bool, "Tail Fraction":dbl}
  T55 = typedef "Phasor.lvlib/Calibration Phasor (m, phi).ctl" = cluster{"m":dbl, "phi":dbl, "Phasor Frequency":dbl[unit], "Reference Lifetime":dbl[unit]}
  T56 = typedef "Phasor.lvlib/Phasor Reference Series.ctl" = cluster{"m Array":dbl[], "phi Array":dbl[], "Phasor Frequency":dbl[unit], "Calibration Lifetime":dbl[unit]}
  T57 = typedef "Phasor.lvlib/Phasor Calibration Map v2.ctl" = cluster{"Phasor Frequency":dbl[unit], "Calibration Lifetime":dbl[unit], "ROI Centers":cluster{"X":i32, "Y":i32}[], "ROI Descriptors":T51[], "Map Resolution X":i32, "Map Resolution Y":i32, "z Array":cdb[]}
  T58 = typedef "Phasor.lvlib/Phasor (g, s).ctl" = cluster{"g":dbl, "s":dbl}
  T59 = typedef "AlliGator Phasor Graph.lvlib/AlliGator Raw Phasor Plot Data v4.ctl" = cluster{"Phasor Plot Name":string, "Raw Phasor Plot":T58[], "Phasor Frequency":dbl[unit], "[Decay Metadata]":T52[], "Raw Phasor Plot SDV":T58[], "Phasor SDV Options":T60, "[Calibration Phasor]":T55[]}
  T60 = typedef "Phasor.lvlib/Phasor Standard Deviation Options.ctl" = cluster{"Compute Estimated SDV":bool, "# Replicas":u32, "Use Estimated Average Phasor":bool}
  T61 = typedef "AlliGator Phasor Plot.lvlib/AlliGator Phasor Multi-Harmonic Data.ctl" = cluster{"Base Frequency":dbl[unit], "# Harmonics":u8, "Harmonic Orders":u8[], "Phasor Plot Settings Checksum":u64, "Phasor Harmonic Data Array":T62[]}
  T62 = typedef "Phasor.lvlib/Phasor Harmonic Data.ctl" = cluster{"Phasor Harmonic Name":string, "Phasor Plot Settings Checksum":u64, "Phasor Frequency":dbl[unit], "Base Frequency":dbl[unit], "Harmonic Order":u8, "Phasor Plot Parameters":string, "Phasor Array [[CSG]]":csg[][], "Dataset File Path":path}
  T63 = typedef "AlliGator Decay Fit Parameter Map.lvlib/AlliGator Decay Fit Options & Parameters v2.ctl" = cluster{"SYNC Period":dbl[unit], "Fit Options":T64, "Fit Parameter Constraints":T71[], "MLE Baseline Offset":dbl, "MLE Baseline Offset Type":T73}
  T64 = typedef "Fits.lvlib/Decay Fit Options v2.ctl" = cluster{"Show Fit Residuals":bool, "Fit Model":T65, "Residual Type":T66, "Max Decay Percentile":dbl, "Min Decay Percentile":dbl, "Show Full Decay":bool, "Weights":T67, "Fitting Method":T68, "Compute Parameter Uncertainties":bool, "Periodic Boundaries":bool, "Model Calculation":T69, "Period":dbl[unit], "Termination Criteria":cluster{"Max Iterations":i32, "Max Function Calls":i32, "Max Time":dbl[unit], "Function Tolerance":dbl, "Parameter Tolerance":dbl, "Gradient Tolerance":dbl, "Min Lambda":dbl, "Max Lambda":dbl, "Initial Tick Count":u32}, "Offset Resolution":dbl[unit], "Use Local IRF":bool, "Fitting Algorithm":T70}
  T65 = typedef "Fits.lvlib/Decay Model.ctl" = enum16{"1-Exponential", "2-Exponentials"}
  T66 = typedef "Fits.lvlib/Residual Type.ctl" = enum16{"Standard", "Normalized", "Reduced"}
  T67 = typedef "Fits.lvlib/Fit Weights Type.ctl" = enum16{"Unweighted", "1/Variance", "Best of All"}
  T68 = typedef "Fits.lvlib/Non-linear Fitting Method v2.ctl" = enum16{"Least Square", "Least Absolute Residual", "Bisquare", "MLE", "-", "Best of All"}
  T69 = typedef "Fits.lvlib/Fit Calculation Method.ctl" = enum16{"Simulation", "Convolution", "Integration"}
  T70 = typedef "Fits.lvlib/Non-linear Fitting Algorithm.ctl" = enum16{"Levenberg-Marquardt", "Trust-Region Dogleg"}
  T71 = typedef "AlliGator Decay Analysis.lvlib/AlliGator Decay Fit.lvlib/AlliGator Decay Fit Parameter Constraints 2.ctl" = cluster{"Fit Parameter":T72, "Min Value":dbl, "Max Value":dbl, "Global":bool, "Used":bool}
  T72 = typedef "Fits.lvlib/Decay Fit Parameters In List.ctl" = enum16{"Offset", "Baseline", "A_1", "tau_1", "A_2", "tau_2"}
  T73 = typedef "Fits.lvlib/MLE Baseline Offset Type.ctl" = enum32{"Absolute", "Percentage"}
  T74 = typedef "Fits.lvlib/Decay Fit Parameters & Derived Quantities List.ctl" = enum16{"Offset", "Baseline", "A_1", "tau_1", "A_2", "tau_2", "<tau>_a", "f1_a", "f2_a", "<tau>_i", "f1_i", "f2_i", "-", "R^2", "Chi^2"}
  T75 = typedef "AlliGator Displayed Image.ctl" = enum16{"Single Gate", "Sum of All Gates", "Max of All Gates", "Min of All Gates", "-", "White Ligth Image", "Mask Image"}
  T76 = typedef "AlliGator Files.lvlib/AlliGator Batch File Conversion Item.ctl" = cluster{"File Path":path, "Saved":bool}
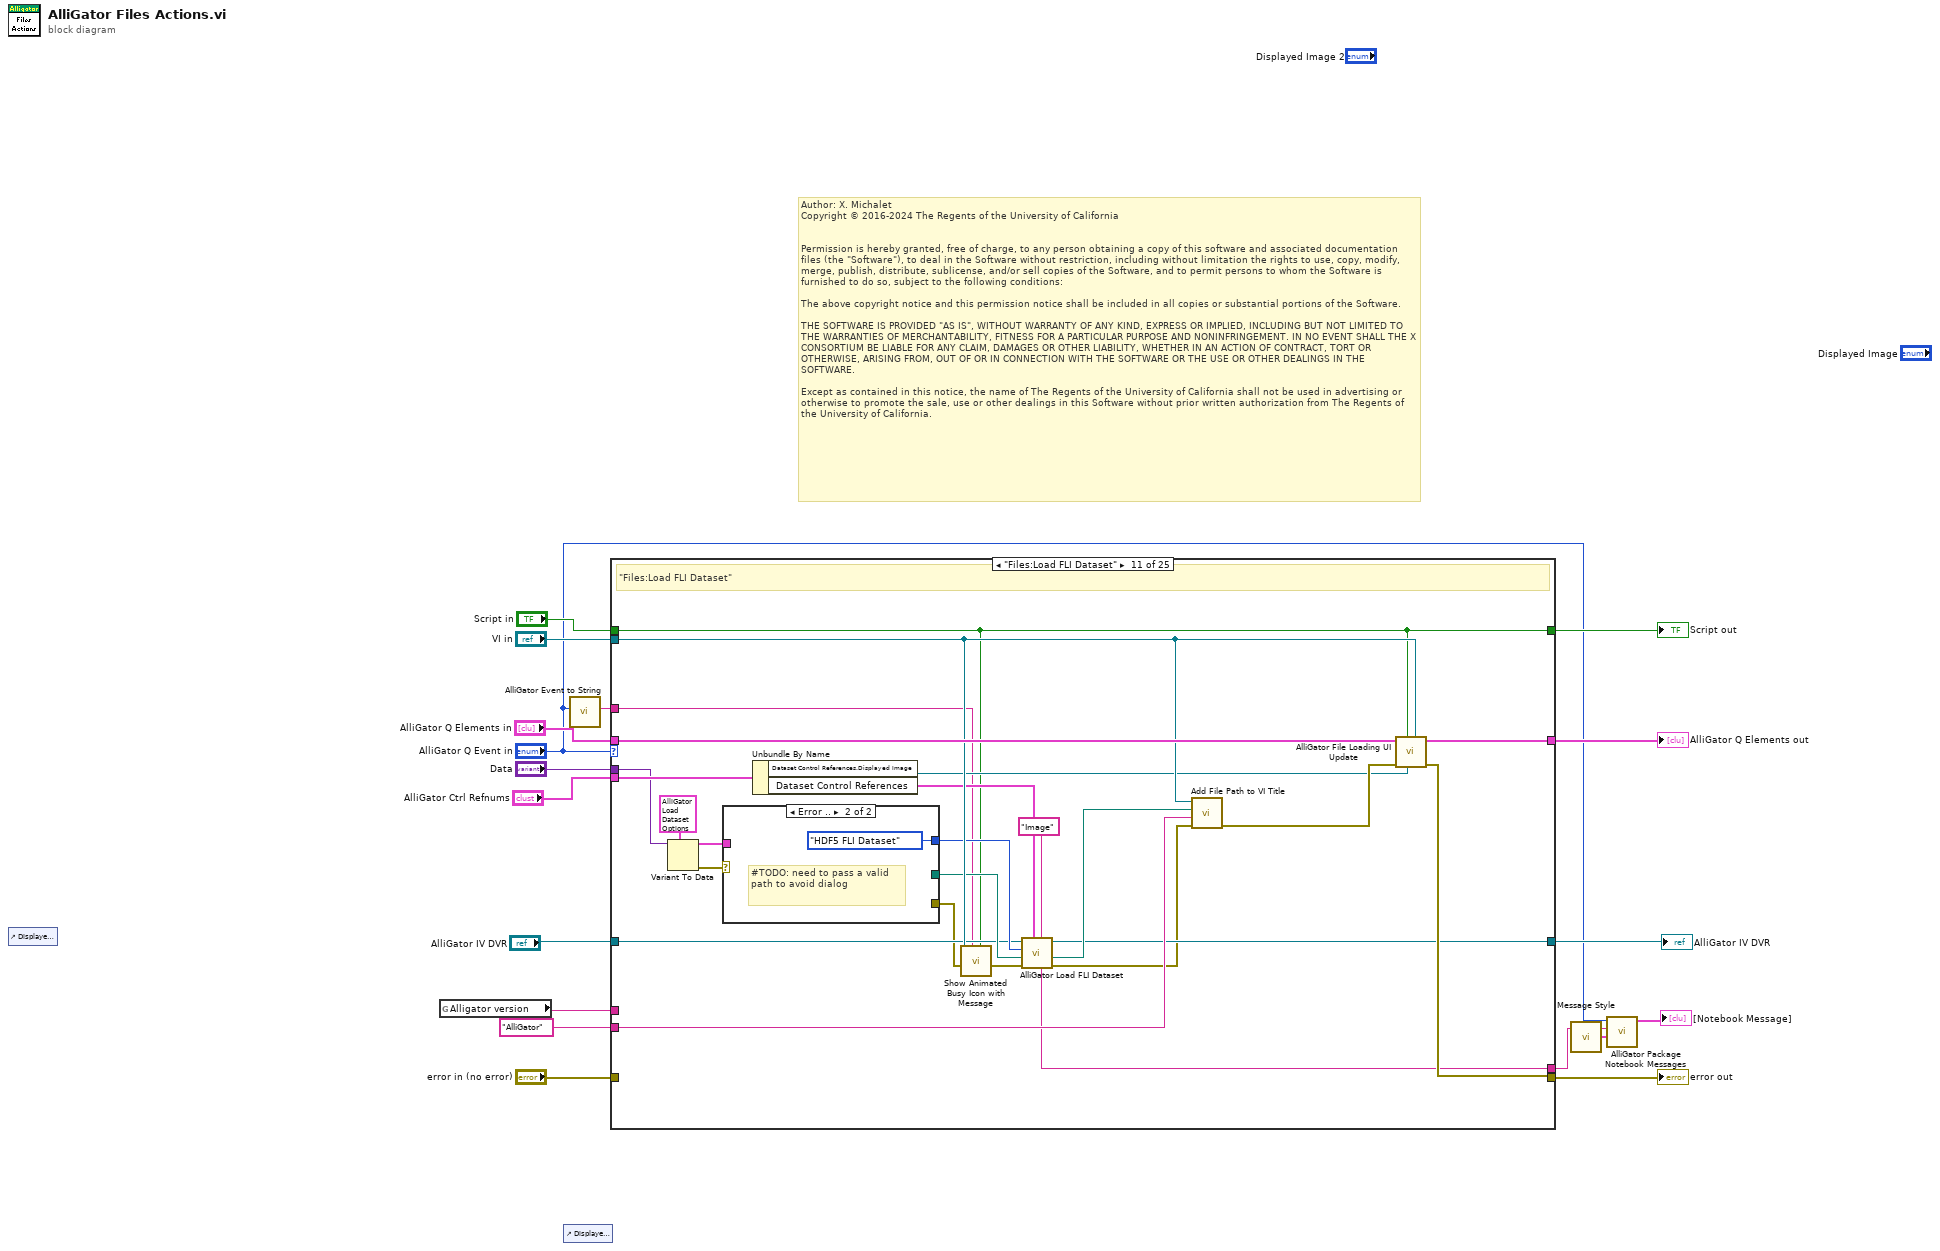
[diagram p0: block diagram]
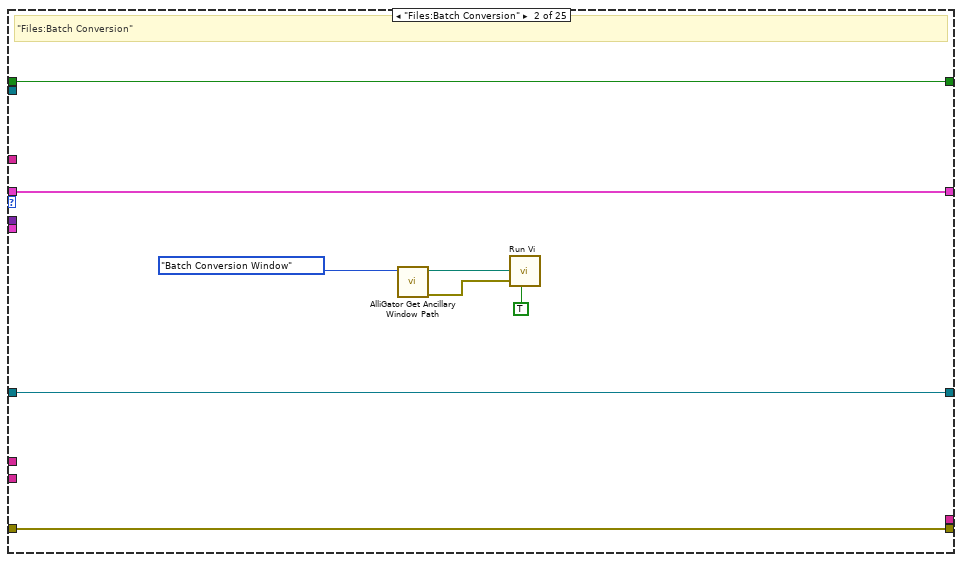
[diagram p3: hidden frame]
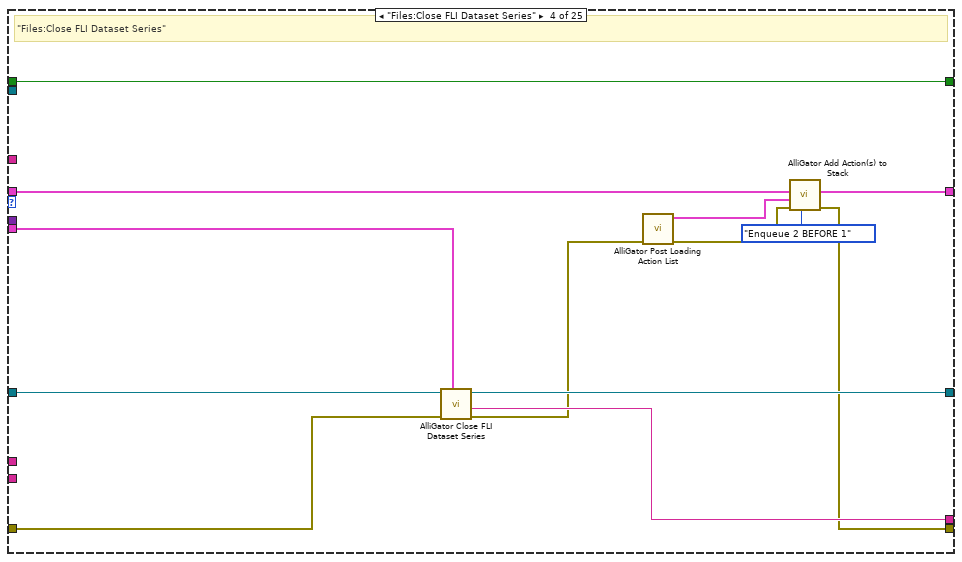
[diagram p5: hidden frame]
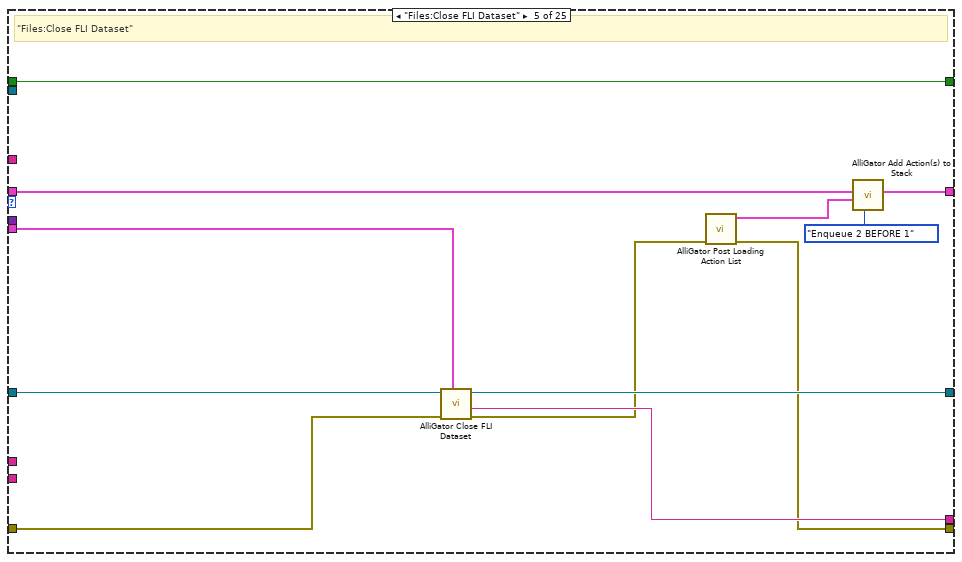
[diagram p6: hidden frame]
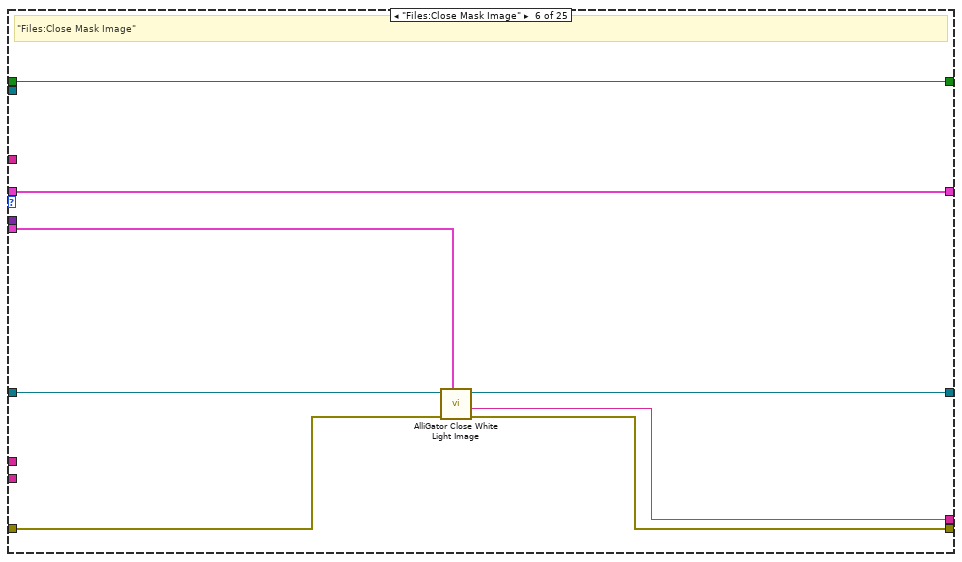
[diagram p7: hidden frame]
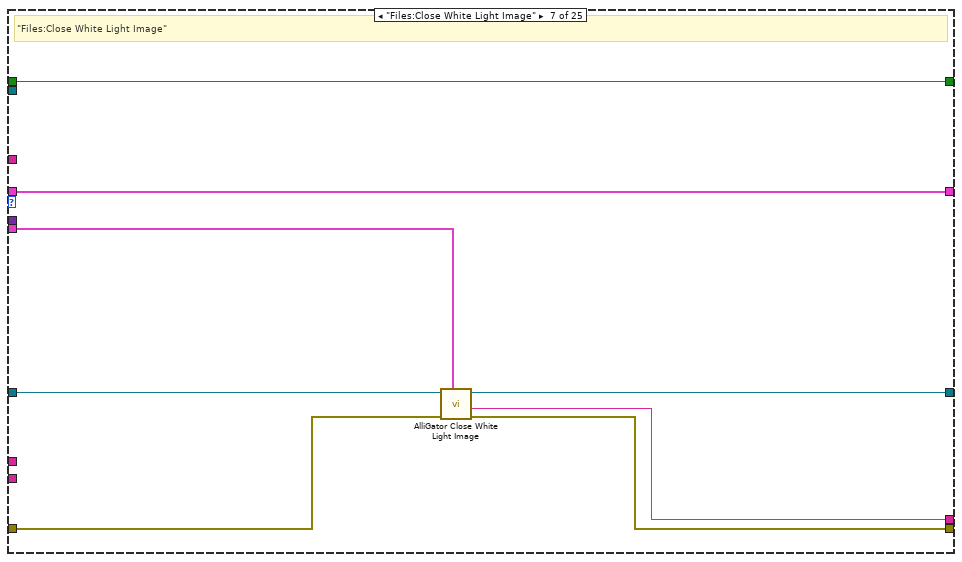
[diagram p8: hidden frame]
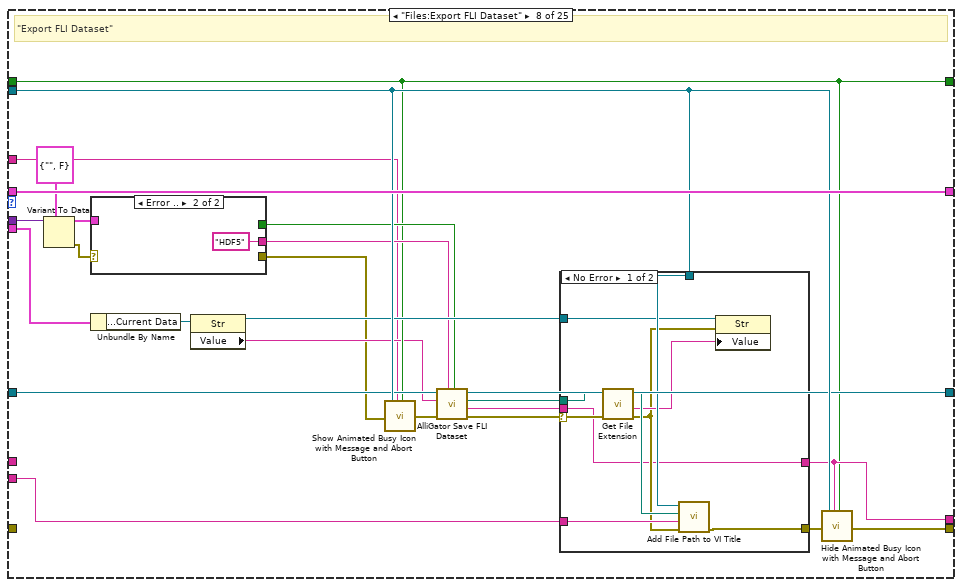
[diagram p9: hidden frame]
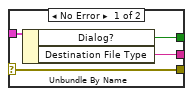
[diagram p10: hidden frame]
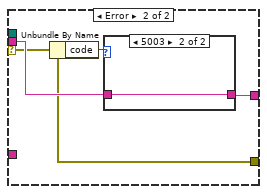
[diagram p11: hidden frame]
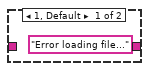
[diagram p12: hidden frame]
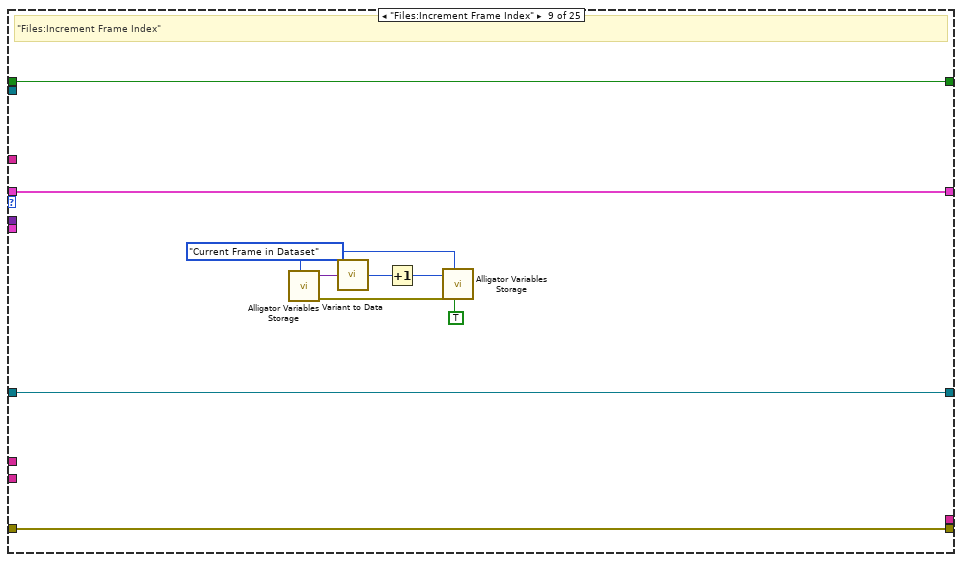
[diagram p13: hidden frame]
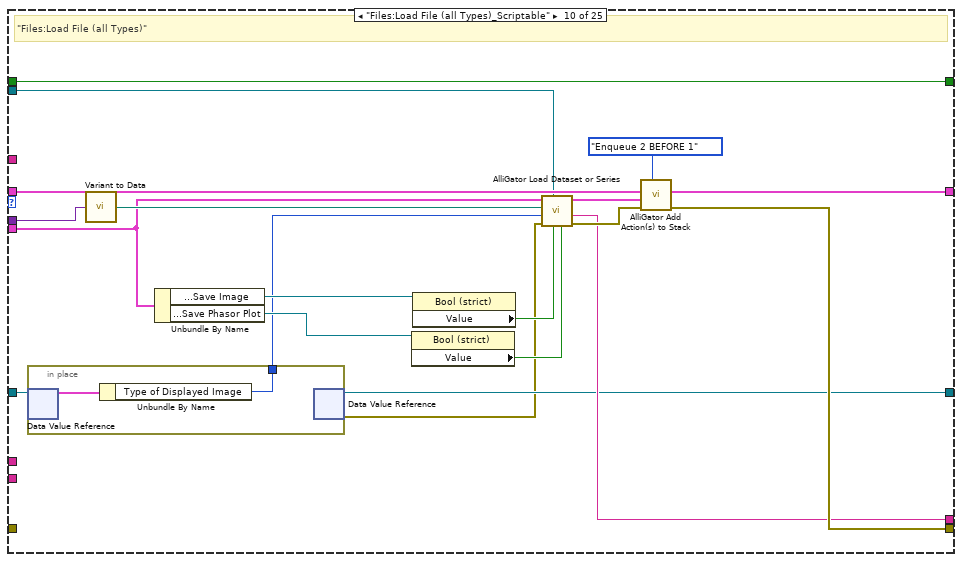
[diagram p14: hidden frame]
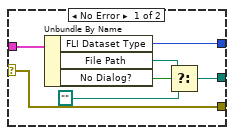
[diagram p15: hidden frame]
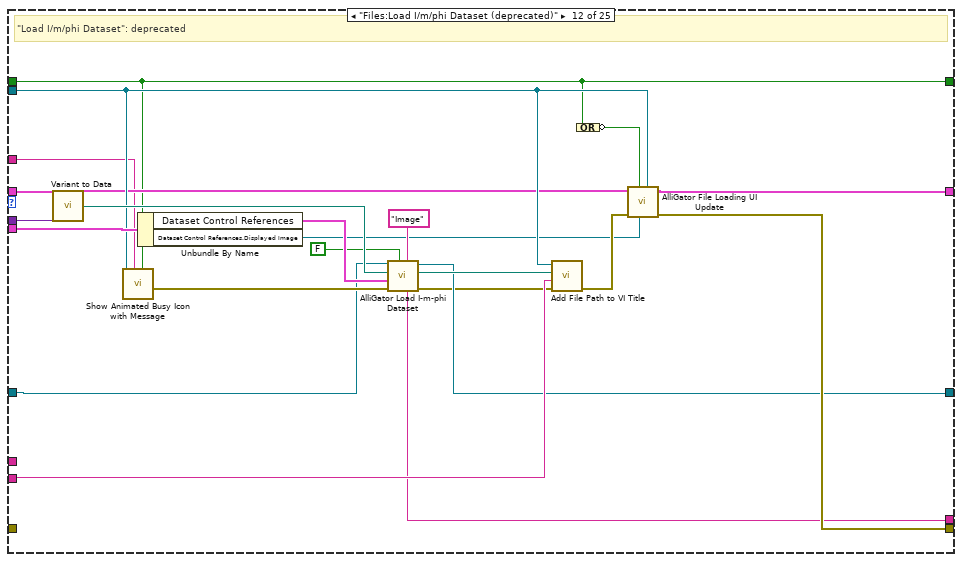
[diagram p16: hidden frame]
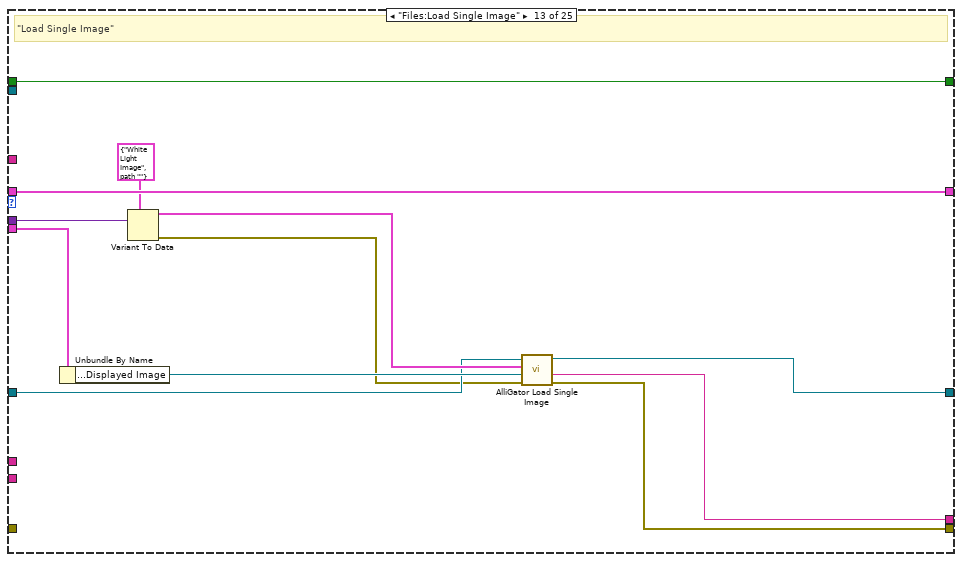
[diagram p17: hidden frame]
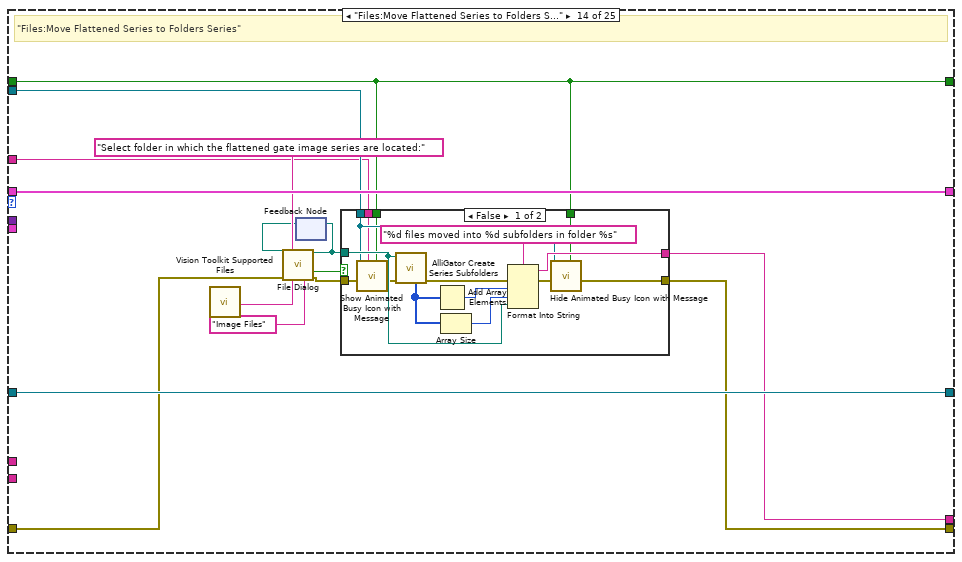
[diagram p18: hidden frame]
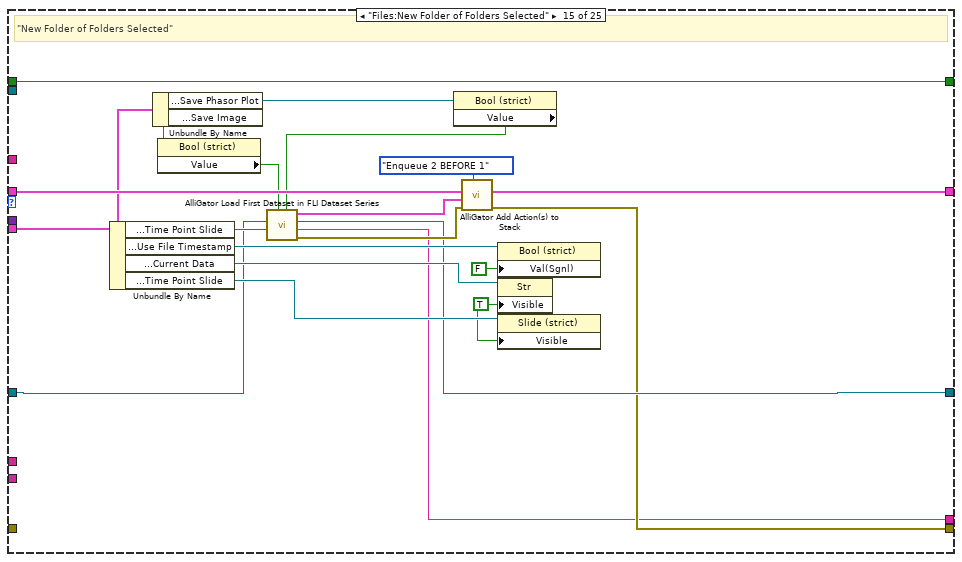
[diagram p20: hidden frame]
diagram:
  # "Author: X. Michalet\nCopyright © 2016-2024 The Regents of the University of California\n \n\nPermission is hereby granted, free of charge, to any person obtaining a copy of this software and associated documentation files (the \"Software\"), to deal in the Software without restriction, including without limitation the rights to use, copy, modify, merge, publish, distribute, sublicense, and/or sell copies of the Software, and to permit persons to whom the Software is furnished to do so, subject to the following conditions:\n\nThe above copyright notice and this permission notice shall be included in all copies or substantial portions of the Software.\n\nTHE SOFTWARE IS PROVIDED \"AS IS\", WITHOUT WARRANTY OF ANY KIND, EXPRESS OR IMPLIED, INCLUDING BUT NOT LIMITED TO THE WARRANTIES OF MERCHANTABILITY, FITNESS FOR A PARTICULAR PURPOSE AND NONINFRINGEMENT. IN NO EVENT SHALL THE X CONSORTIUM BE LIABLE FOR ANY CLAIM, DAMAGES OR OTHER LIABILITY, WHETHER IN AN ACTION OF CONTRACT, TORT OR OTHERWISE, ARISING FROM, OUT OF OR IN CONNECTION WITH THE SOFTWARE OR THE USE OR OTHER DEALINGS IN THE SOFTWARE.\n\nExcept as contained in this notice, the name of The Regents of the University of California shall not be used in advertising or otherwise to promote the sale, use or other dealings in this Software without prior written authorization from The Regents of the University of California."
  n1 = control-ref of="Displayed Image 2"() -> ()  [unwired: 1 out]
  n2 = global read "AlliGator Globals.vi" "Alligator version"() -> (w10:string)
  n3 = control-ref of="Displayed Image"() -> ()  [unwired: 1 out]
  n4 = call "AlliGator Event to String.vi"("AlliGator Q Event"="AlliGator Q Event in") -> ("String"=w6:string)  [unwired: 8 in]
  n5 = case shown="\"Files:Load FLI Dataset\"" "AlliGator Q Event in" {
    tunnel: "Data" -> [_ _ _ _ _ _ _ w96 _ w143 w169 w208 w220 _ _ w299 _ w373 _ _ w413 w444 w461 w469 w486]
    tunnel: "AlliGator Q Elements in" -> [w22 w30 w34 w39 w53 w67 w75 w100 w131 w150 w177 w194 w218 w235 w270 w301 w345 w368 w390 w399 w418 w447 w463 w471 w487]
    tunnel: [w22 w30 w34 w38 w52 w67 w75 w100 w131 w148 w176 w202 w218 w235 w268 w300 w343 w366 w388 w399 w417 w447 w463 w471 w487] -> w12
    tunnel: "VI in" -> [_ _ _ _ _ _ _ w95 _ w136 w172 w196 _ w225 _ _ _ _ _ _ w414 _ _ _ w480]
    tunnel: w10 -> [_ _ _ _ _ _ _ _ _ _ _ _ _ _ _ _ _ _ _ _ _ _ _ _ _]
    tunnel: [w21 w29 w33 w47 w59 w66 w74 w80 w130 w151 w156 w187 w219 w224 w272 w295 w346 w374 w392 w398 w415 w446 w462 w470 w473] -> w13
    tunnel: "Script in" -> [w21 w29 w33 w47 w59 w66 w74 w80 w130 w151 w156 w187 w219 w224 w272 w295 w346 w374 w392 w398 w415 w446 w462 w470 w473]
    tunnel: "AlliGator" ("Sender") -> [_ _ _ _ _ _ _ w99 _ _ w174 w199 _ _ _ _ _ _ _ _ w411 _ _ _ _]
    tunnel: "error in (no error)" -> [w20 w28 w32 w44 w56 w62 w70 _ w129 _ _ _ _ w227 _ _ _ _ _ w394 _ w445 _ _ _]
    tunnel: [w20 w28 w32 w37 w49 w63 w71 w98 w129 w146 w175 w201 w211 w228 w253 w280 w341 w364 w386 w395 w410 w445 w456 w465 w481] -> w5
    tunnel: "AlliGator Ctrl Refnums" -> [_ _ _ w43 w55 w61 w69 w97 _ w141 w173 w198 w215 _ w264 w289 _ w358 _ _ _ _ _ _ _]
    tunnel: "AlliGator IV DVR" -> [w19 w23 w31 w46 w58 w65 w73 w85 w128 w135 w161 w192 w212 w234 w254 w276 w339 w351 w384 w397 w404 w437 w455 w464 w477]
    tunnel: [w19 w23 w31 w45 w57 w64 w72 w82 w128 w134 w160 w191 w213 w234 w255 w275 w339 w350 w384 w396 w405 w437 w455 w464 w478] -> w7
    tunnel: w6 -> [_ _ _ _ _ _ _ w76 _ _ w158 w189 _ w223 _ _ _ _ _ _ _ _ _ _ w475]
    tunnel: [_ _ _ w42 w54 w60 w68 w94 _ w140 w157 w188 w209 w226 w252 w279 _ _ _ w393 _ _ _ _ w474] -> w3
    frame "---- Files ----", Default {
    }
    frame "Files:Batch Conversion" {
      # "\"Files:Batch Conversion\""
      n6 = call "AlliGator Get Ancillary Window Path.vi"("AlliGator Window"=AlliGator_Windows_List."Batch Conversion Window" ("AlliGator Windows")) -> ("Error Out"=w26:errorcluster, "VI Path"=w27:path)  [unwired: 9 in]
      n7 = call "Run Vi.vi"("VI Path"=w27, "error in (no error)"=w26, "Start Hidden? (F)"=TRUE) -> ()  [unwired: 5 in, 2 out]
    }
    frame "Files:Check #Frames in Dataset" {
      # "#TODO"
      # "\"Files:Check #Frames in Dataset\""
    }
    frame "Files:Close FLI Dataset Series" {
      # "\"Files:Close FLI Dataset Series\""
      n8 = call "AlliGator Close FLI Dataset Series.vi"("AlliGator Ctrl Refnums"=w43, "error in (no error)"=w44, "AlliGator IV DVR in"=w46) -> ("error out"=w36:errorcluster, "Message"=w42:string, "AlliGator IV DVR out"=w45:refnum<data-value>)  [unwired: 6 in]
      n9 = call "AlliGator Post Loading Action List.vi"("Error In"=w36) -> ("Error Out"=w35:errorcluster, "Action List"=w41:T5[])  [unwired: 9 in]
      n10 = call-poly "AlliGator Add Action(s) to Stack.vi"("Elements Order in Action Stack (Default: 2 BEFORE 1)"=Alligator_Elements_Order_in_Action_Stack."Enqueue 2 BEFORE 1", "Error In"=w35, "Alligator Queue Element 2"=w41, "Alligator Queue Element 1"=w39) -> ("Error Out"=w37:errorcluster, "Alligator Queue Element 1 (+ 2)"=w38:T5[])  [unwired: 6 in]
    }
    frame "Files:Close FLI Dataset" {
      # "\"Files:Close FLI Dataset\""
      n11 = call "AlliGator Close FLI Dataset.vi"("AlliGator Ctrl Refnums"=w55, "error in (no error)"=w56, "AlliGator IV DVR in"=w58) -> ("error out"=w50:errorcluster, "Message"=w54:string, "AlliGator IV DVR out"=w57:refnum<data-value>)  [unwired: 6 in]
      n12 = call "AlliGator Post Loading Action List.vi"("Error In"=w50) -> ("Error Out"=w49:errorcluster, "Action List"=w51:T5[])  [unwired: 9 in]
      n13 = call-poly "AlliGator Add Action(s) to Stack.vi"("Elements Order in Action Stack (Default: 2 BEFORE 1)"=Alligator_Elements_Order_in_Action_Stack."Enqueue 2 BEFORE 1", "Alligator Queue Element 2"=w51, "Alligator Queue Element 1"=w53) -> ("Alligator Queue Element 1 (+ 2)"=w52:T5[])  [unwired: 7 in, 1 out]
    }
    frame "Files:Close Mask Image" {
      # "\"Files:Close Mask Image\""
      n14 = call "AlliGator Close White Light Image.vi"("AlliGator Ctrl Refnums"=w61, "error in (no error)"=w62, "AlliGator IV DVR in"=w65) -> ("error out"=w63:errorcluster, "Message"=w60:string, "AlliGator IV DVR out"=w64:refnum<data-value>)  [unwired: 6 in]
    }
    frame "Files:Close White Light Image" {
      # "\"Files:Close White Light Image\""
      n15 = call "AlliGator Close White Light Image.vi"("AlliGator Ctrl Refnums"=w69, "error in (no error)"=w70, "AlliGator IV DVR in"=w73) -> ("error out"=w71:errorcluster, "Message"=w68:string, "AlliGator IV DVR out"=w72:refnum<data-value>)  [unwired: 6 in]
    }
    frame "Files:Export FLI Dataset" {
      # "\"Export FLI Dataset\""
      n16 = Variant To Data(type=T17 {"Destination File Type"="", "Dialog?"=FALSE} ("output cluster"), Variant=w96) -> (data=w88:T17, error out=w78:errorcluster)  [unwired: 1 in]
      n17 = case shown="Error .." w78 {
        selector: w78 -> [w101 _]
        tunnel: w88 -> [w104 _]
        tunnel: [w103 "HDF5" ("Destination File Type")] -> w84
        tunnel: [w102 _] -> w83
        tunnel: [w101 _] -> w77
        frame No Error {
          n18 = Unbundle By Name(w104) -> ("Dialog?"=w102:bool, "Destination File Type"=w103:string)
        }
        frame Error {
        }
      }
      n19 = Unbundle By Name(w97) -> ("Dataset Control References.Current Data"=w89:refnum<vi>)
      n20 = property class="Str"(reference=w89) -> (reference out=w87:refnum<vi>, "Value"=w79:string)  [unwired: 1 in, 1 out]
      n21 = call "Show Animated Busy Icon with Message and Abort Button.vi"("Already active? (F)"=w80, "Message"=w76, "Target VI reference"=w95, "Error In"=w77) -> ("Error Out"=w81:errorcluster)  [unwired: 15 in]
      n22 = call "AlliGator Save FLI Dataset.vi"("Dialog?"=w83, "Destination File Type"=w84, "error in"=w81, "Current Data"=w79, "AlliGator IV DVR"=w85) -> ("error out"=w93:errorcluster, "Output String"=w91:string, "File Path out"=w90:path, "AlliGator IV DVR"=w82:refnum<data-value>)  [unwired: 3 in]
      n23 = case shown="No Error" w93 {
        selector: w93 -> [w111 w116]
        tunnel: [w110 w116] -> w92
        tunnel: w91 -> [w106 w119]
        tunnel: w90 -> [w114 _]
        tunnel: w95 -> [w115 _]
        tunnel: w99 -> [w113 _]
        tunnel: [w106 w117] -> w94
        tunnel: w87 -> [w109 _]
        frame No Error {
          n24 = call <vilib>:"Get File Extension.vi"("error in (no error)"=w111, "file"=w114) -> ("error out"=w107:errorcluster, "filename without extension"=w108:string, "dup file"=w112:path)  [unwired: 5 in, 2 out]
          n25 = call "Add File Path to VI Title.vi"("Error In"=w107, "VI Title"=w113, "File Path"=w112, "VI Refnum"=w115) -> ("Error Out"=w110:errorcluster)  [unwired: 7 in]
          n26 = property class="Str"(reference=w109, error in=w107, "Value"=w108) -> ()  [unwired: 2 out]
        }
        frame Error {
          n27 = Unbundle By Name(w116) -> ("code"=w118:i32)
          n28 = case shown="5003" w118 {
            tunnel: ["Error loading file..." ("Message") w121] -> w117
            tunnel: w119 -> [_ w121]
            frame 1, Default {
            }
            frame 5003 {
            }
          }
        }
      }
      n29 = call "Hide Animated Busy Icon with Message and Abort Button.vi"("Already active? (F)"=w80, "Message"=w94, "Target VI reference"=w95, "Error In"=w92) -> ("Error Out"=w98:errorcluster)  [unwired: 15 in]
    }
    frame "Files:Increment Frame Index" {
      w125 = AlliGator_Variables_List."Current Frame in Dataset" ("Alligator Variable")
      # "\"Files:Increment Frame Index\""
      n30 = call "Alligator Variables Storage.vi"("AlliGator Variable"=w125) -> ("Error Out"=w126:errorcluster, "Data out"=w127:variant)  [unwired: 8 in, 1 out]
      n31 = call-poly "Variant to Data.vi"("Variant"=w127) -> ("Value"=w124:i32)  [unwired: 8 in]
      n32 = Increment(x=w124) -> (x+1=w123:i32)
      n33 = call "Alligator Variables Storage.vi"("Get(F)/Set"=TRUE, "AlliGator Variable"=w125, "Error In"=w126, "Data in"=w123) -> ()  [unwired: 5 in, 3 out]
    }
    frame "Files:Load File (all Types)_Scriptable" {
      # "\"Files:Load File (all Types)\""
      n34 = in-place {
        in-place-border: [w152] -> w132
        n35 = in-place-dvr #1(w135) -> (w153:T45)  [unwired: 1 out]
        n36 = Unbundle By Name(w153) -> ("Type of Displayed Image"=w152:T1)
        n37 = in-place-dvr #1() -> (w134:refnum<data-value>, w133:errorcluster)  [unwired: 1 in]
      }
      n38 = call-poly "Variant to Data.vi"("Variant"=w143) -> ("Path"=w142:path)  [unwired: 8 in]
      n39 = Unbundle By Name(w141) -> ("Dataset Control References.Save Image"=w144:refnum<vi>, "Phasor Plot Ctrl Refnums.Save Phasor Plot"=w138:refnum<vi>)
      n40 = property class="Bool (strict)"(reference=w138) -> ("Value"=w137:bool)  [unwired: 1 in, 2 out]
      n41 = property class="Bool (strict)"(reference=w144) -> ("Value"=w139:bool)  [unwired: 1 in, 2 out]
      n42 = call "AlliGator Load Dataset or Series.vi"("Save Phasor Plot with Overlay"=w137, "Save Image with Overlay"=w139, "VI in"=w136, "error in (no error)"=w133, "Type of Displayed Image"=w132, "File/Folder Path"=w142, "AlliGator Ctrl Refnums"=w141) -> ("error out"=w147:errorcluster, "Message"=w140:string, "AlliGator Q Elements out"=w149:T5[])  [unwired: 2 in]
      n43 = call-poly "AlliGator Add Action(s) to Stack.vi"("Elements Order in Action Stack (Default: 2 BEFORE 1)"=Alligator_Elements_Order_in_Action_Stack."Enqueue 2 BEFORE 1", "Error In"=w147, "Alligator Queue Element 2"=w149, "Alligator Queue Element 1"=w150) -> ("Error Out"=w146:errorcluster, "Alligator Queue Element 1 (+ 2)"=w148:T5[])  [unwired: 6 in]
    }
    frame "Files:Load FLI Dataset" {
      # "\"Files:Load FLI Dataset\""
      n44 = Variant To Data(type=T18 {"FLI Dataset Type"=enum."HDF5 FLI Dataset", "No Dialog?"=FALSE, "File Path"=path ""} ("output cluster"), Variant=w169) -> (data=w168:T18, error out=w155:errorcluster)  [unwired: 1 in]
      n45 = case shown="Error .." w155 {
        selector: w155 -> [w179 _]
        tunnel: w168 -> [w185 _]
        tunnel: [w182 AlliGator_FLI_Dataset_Type."HDF5 FLI Dataset" ("FLI Dataset Type")] -> w166
        tunnel: [w180 _] -> w164
        tunnel: [w179 _] -> w154
        frame No Error {
          n46 = Unbundle By Name(w185) -> ("FLI Dataset Type"=w182:T19, "File Path"=w181:path, "No Dialog?"=w184:bool)
          n47 = Select(t=w181, s=w184, f=path "") -> (s? t:f=w180:path)
        }
        frame Error {
          # "#TODO: need to pass a valid path to avoid dialog"
        }
      }
      n48 = Unbundle By Name(w173) -> ("Dataset Control References.Displayed Image"=w171:refnum<vi>, "Dataset Control References"=w167:T11)
      n49 = call "Show Animated Busy Icon with Message.vi"("Already active? (F)"=w156, "Message"=w158, "Error In"=w154, "Target VI Refnum"=w172) -> ("Error Out"=w165:errorcluster)  [unwired: 7 in]
      n50 = call "AlliGator Load FLI Dataset.vi"("Image Type"="Image", "Dataset Control References"=w167, "error in"=w165, "Single Data Point Path"=w164, "FLI Dataset Type"=w166, "AlliGator IV DVR in"=w161) -> ("error out"=w159:errorcluster, "File Path out"=w163:path, "AlliGator IV DVR out"=w160:refnum<data-value>, "Message"=w157:string)  [unwired: 2 in]
      n51 = call "Add File Path to VI Title.vi"("Error In"=w159, "VI Title"=w174, "File Path"=w163, "VI Refnum"=w172) -> ("Error Out"=w178:errorcluster)  [unwired: 7 in]
      n52 = call "AlliGator File Loading UI Update.vi"("VI in"=w172, "Displayed Image"=w171, "Busy Icon already active?"=w156, "error in (no error)"=w178, "Alligator Queue Elements in"=w177) -> ("error out"=w175:errorcluster, "Alligator Queue Elements out"=w176:T5[])  [unwired: 5 in]
    }
    frame "Files:Load I/m/phi Dataset (deprecated)" {
      # "\"Load I/m/phi Dataset\": deprecated"
      n53 = call-poly "Variant to Data.vi"("Variant"=w208) -> ("Path"=w206:path)  [unwired: 8 in]
      n54 = call "Show Animated Busy Icon with Message.vi"("Already active? (F)"=w187, "Message"=w189, "Target VI Refnum"=w196) -> ("Error Out"=w205:errorcluster)  [unwired: 8 in]
      n55 = Unbundle By Name(w198) -> ("Dataset Control References"=w197:T11, "Dataset Control References.Displayed Image"=w195:refnum<vi>)
      n56 = call "AlliGator Load I-m-phi Dataset.vi"("Image Type"="Image", "Bkgd Image Subtraction?"=FALSE, "error in (no error)"=w205, "Control References"=w197, "Folder Path"=w206, "AlliGator IV DVR in"=w192) -> ("error out"=w190:errorcluster, "Folder Path (dup)"=w200:path, "AlliGator IV DVR out"=w191:refnum<data-value>, "Result String"=w188:string)  [unwired: 2 in]
      n57 = call "Add File Path to VI Title.vi"("Error In"=w190, "VI Title"=w199, "File Path"=w200, "VI Refnum"=w196) -> ("Error Out"=w203:errorcluster)  [unwired: 7 in]
      n58 = Compound Arithmetic op=OR(w187) -> (invert w204:bool)
      n59 = call "AlliGator File Loading UI Update.vi"("VI in"=w196, "Displayed Image"=w195, "Busy Icon already active?"=w204, "error in (no error)"=w203, "Alligator Queue Elements in"=w194) -> ("error out"=w201:errorcluster, "Alligator Queue Elements out"=w202:T5[])  [unwired: 5 in]
    }
    frame "Files:Load Single Image" {
      # "\"Load Single Image\""
      n60 = Unbundle By Name(w215) -> ("Dataset Control References.Displayed Image"=w214:refnum<vi>)
      n61 = Variant To Data(type=T20 {"Image Type"=enum."White Light Image", "Image Path"=path ""}, Variant=w220) -> (data=w216:T20, error out=w210:errorcluster)  [unwired: 1 in]
      n62 = call "AlliGator Load Single Image.vi"("error in (no error)"=w210, "Displayed Image refnum"=w214, "Single Image File Info"=w216, "AlliGator Internal Data DVR"=w212) -> ("error out"=w211:errorcluster, "Message"=w209:string, "AlliGator Internal Data DVR"=w213:refnum<data-value>)  [unwired: 5 in]
    }
    frame "Files:Move Flattened Series to Folders Series" {
      # "\"Files:Move Flattened Series to Folders Series\""
      n63 = call "Vision Toolkit Supported Files.vi"() -> ("Pattern String"=w232:string)  [unwired: 7 in, 1 out]
      n64 = feedback #2() -> (w222:path)  [unwired: 1 in]
      n65 = call "File Dialog"("start path"=w222, "prompt"="Select folder in which the flattened gate image series are located:", "error in"=w227, "pattern (all files)"=w232, "pattern label"="Image Files") -> ("selected path"=w221:path, "cancelled"=w229:bool, "error out"=w230:errorcluster)  [unwired: 7 in, 1 out]
      n66 = feedback-in #2(w221) -> ()
      n67 = case shown="False" w229 {
        tunnel: w221 -> [w242 _]
        tunnel: w230 -> [w250 w251]
        tunnel: [w240 w251] -> w228
        tunnel: [w247 _] -> w226
        tunnel: w225 -> [w239 _]
        tunnel: w224 -> [w238 _]
        tunnel: w224 -> [w237 _]
        tunnel: w223 -> [w236 _]
        frame False {
          n68 = call "Show Animated Busy Icon with Message.vi"("Already active? (F)"=w238, "Message"=w236, "Error In"=w250, "Target VI Refnum"=w239) -> ("Error Out"=w241:errorcluster)  [unwired: 7 in]
          n69 = call "AlliGator Create Series Subfolders.vi"("error in (no error)"=w241, "Path"=w242) -> ("error out"=w249:errorcluster, "# Files"=w245:i32[])  [unwired: 3 in, 5 out]
          n70 = Add Array Elements(numeric array=w245) -> (sum=w244:i32)
          n71 = Array Size(array=w245) -> (size(s)=w246:i32)
          n72 = Format Into String(format string="%d files moved into %d subfolders in folder %s", error in=w249, w244, w246, w242) -> (resulting string=w247:string, error out=w248:errorcluster)  [unwired: 1 in]
          n73 = call "Hide Animated Busy Icon with Message.vi"("Already active? (F)"=w237, "Error In"=w248, "Target VI reference"=w239) -> ("Error Out"=w240:errorcluster)  [unwired: 8 in]
        }
        frame True {
        }
      }
    }
    frame "Files:New Folder of Folders Selected" {
      w256 = TRUE ("Get(F)/Set")
      # "\"New Folder of Folders Selected\""
      n74 = Unbundle By Name(w264) -> ("Dataset Control References.Time Point Slide"=w271:refnum<vi>, "Other AlliGator Ctrl Refnums.Use File Timestamp"=w260:refnum<vi>, "Dataset Control References.Current Data"=w258:refnum<vi>, "Dataset Control References.Time Point Slide"=w257:refnum<vi>)
      n75 = Unbundle By Name(w264) -> ("Phasor Plot Ctrl Refnums.Save Phasor Plot"=w265:refnum<vi>, "Dataset Control References.Save Image"=w262:refnum<vi>)
      n76 = property class="Bool (strict)"(reference=w262) -> ("Value"=w261:bool)  [unwired: 1 in, 2 out]
      n77 = property class="Bool (strict)"(reference=w265) -> ("Value"=w263:bool)  [unwired: 1 in, 2 out]
      n78 = call "AlliGator Load First Dataset in FLI Dataset Series.vi"("Save Phasor Plot with Overlay"=w263, "Save Image with Overlay"=w261, "Time Slider Refnum"=w271, "AlliGator IV DVR in"=w254) -> ("Error Out"=w267:errorcluster, "Message"=w252:string, "AlliGator IV DVR out"=w255:refnum<data-value>, "Alligator Queue Elements out"=w269:T5[])  [unwired: 4 in]
      n79 = call-poly "AlliGator Add Action(s) to Stack.vi"("Elements Order in Action Stack (Default: 2 BEFORE 1)"=Alligator_Elements_Order_in_Action_Stack."Enqueue 2 BEFORE 1", "Error In"=w267, "Alligator Queue Element 2"=w269, "Alligator Queue Element 1"=w270) -> ("Error Out"=w253:errorcluster, "Alligator Queue Element 1 (+ 2)"=w268:T5[])  [unwired: 6 in]
      n80 = property class="Bool (strict)"(reference=w260, "Val(Sgnl)"=FALSE ("Value (Signaling)")) -> ()  [unwired: 1 in, 2 out]
      n81 = property class="Str"(reference=w258, "Visible"=w256) -> ()  [unwired: 1 in, 2 out]
      n82 = property class="Slide (strict)"(reference=w257, "Visible"=w256) -> ()  [unwired: 1 in, 2 out]
    }
    frame "Files:New Folder Selected" {
      # "\"New Folder Selected\""
      n83 = in-place {
        in-place-border: [w306] -> w283
        in-place-border: [w305] -> w282
        in-place-border: [w304] -> w281
        in-place-border: [w302] -> w273
        n84 = in-place-dvr #3(w276) -> (w303:T45)  [unwired: 1 out]
        n85 = Unbundle By Name(w303) -> ("Current Dataset"=w302:i32, "Single Data Point Path"=w306:path, "Single Dataset Type"=w305:T19, "[Time-Series Paths]"=w304:path[])
        n86 = in-place-dvr #3() -> (w275:refnum<data-value>, w274:errorcluster)  [unwired: 1 in]
      }
      n87 = Unbundle By Name(w289) -> ("Phasor Plot Ctrl Refnums.Save Phasor Plot"=w287:refnum<vi>, "Dataset Control References.Save Image"=w285:refnum<vi>, "Dataset Control References.Displayed Image"=w278:refnum<vi>)
      n88 = call-poly "Variant to Data.vi"("Variant"=w299) -> ("Path"=w298:path)  [unwired: 8 in]
      n89 = property class="Bool (strict)"(reference=w287) -> ("Value"=w286:bool)  [unwired: 1 in, 2 out]
      n90 = property class="Bool (strict)"(reference=w285) -> ("Value"=w284:bool)  [unwired: 1 in, 2 out]
      n91 = property class="Enum (strict)"(reference=w278) -> ("Value"=w277:T75)  [unwired: 1 in, 2 out]
      n92 = Empty Array?(array=w281) -> (empty?=w296:bool)
      n93 = call "AlliGator Update Data File.vi"("Error In"=w274, "Single Data Point Path"=w283, "New File Path in"=w298) -> ("Error Out"=w291:errorcluster, "Update Data File?"=w290:bool, "File Path out"=w293:path)  [unwired: 6 in]
      n94 = Path To String(path=w293) -> (string=w297:string)
      n95 = case shown="True" w290 {
        tunnel: w301 -> [w308 w315]
        tunnel: [w308 w314] -> w300
        tunnel: w293 -> [_ w321]
        tunnel: w291 -> [w307 w320]
        tunnel: w282 -> [_ w319]
        tunnel: w286 -> [_ w318]
        tunnel: w284 -> [_ w317]
        tunnel: [w307 w311] -> w288
        tunnel: w277 -> [_ w310]
        tunnel: w273 -> [_ w309]
        frame False {
        }
        frame True {
          n96 = call "AlliGator Script_Open Single FLI Dataset.vi"("Type of Displayed Image"=w310, "FLI Dataset Type"=w319, "File Path"=w321, "Dataset index in Series (0)"=w309, "Save Image with Overlay"=w318, "Error In"=w320, "Save Phasor Plot with Overlay"=w317) -> ("Action List out"=w316:T5[], "Error Out"=w312:errorcluster)  [unwired: 7 in]
          n97 = call-poly "AlliGator Add Action(s) to Stack.vi"("Elements Order in Action Stack (Default: 2 BEFORE 1)"=Alligator_Elements_Order_in_Action_Stack."Enqueue 2 BEFORE 1", "Error In"=w312, "Alligator Queue Element 2"=w316, "Alligator Queue Element 1"=w315) -> ("Error Out"=w311:errorcluster, "Alligator Queue Element 1 (+ 2)"=w314:T5[])  [unwired: 6 in]
        }
      }
      n98 = File/Directory Info(path=w293, error in=w288) -> (directory=w294:bool, error out=w292:errorcluster)  [unwired: 5 out]
      n99 = case shown="\"New Path\", Default" w297 {
        selector: w297 -> [_ w328]
        tunnel: w296 -> [_ w327]
        tunnel: w294 -> [_ w326]
        tunnel: w292 -> [w322 w325]
        tunnel: [w322 w324] -> w280
        tunnel: [_ w323] -> w279
        frame "" {
        }
        frame "New Path", Default {
          n100 = case shown="True" w327 {
            tunnel: w328 -> [_ w338]
            tunnel: w326 -> [_ w336]
            tunnel: w325 -> [w329 w332]
            tunnel: [w329 w330] -> w324
            tunnel: [_ w331] -> w323
            frame False {
            }
            frame True {
              n101 = Select(t="Folder" ("input 1"), s=w336, f="File" ("input 1")) -> (s? t:f=w334:string)
              n102 = Format Into String(format string="New %s Selected: %s" ("initial string"), error in=w332, w334, w338) -> (resulting string=w331:string, error out=w330:errorcluster)  [unwired: 1 in]
            }
          }
        }
      }
    }
    frame "Files:Open Mask Image" {
      # "\"Open Mask Image\""
      n103 = call "AlliGator Script Open Mask Image.vi"() -> ("Error Out"=w342:errorcluster, "Action List out"=w344:T5[])  [unwired: 10 in]
      n104 = call-poly "AlliGator Add Action(s) to Stack.vi"("Elements Order in Action Stack (Default: 2 BEFORE 1)"=Alligator_Elements_Order_in_Action_Stack."Enqueue 2 BEFORE 1", "Error In"=w342, "Alligator Queue Element 2"=w344, "Alligator Queue Element 1"=w345) -> ("Error Out"=w341:errorcluster, "Alligator Queue Element 1 (+ 2)"=w343:T5[])  [unwired: 6 in]
    }
    frame "Files:Open Single Dataset" {
      w355 = FALSE  # Single Dataset
      # "If loading fails, we lose this information!"
      # "\"Files:Open Single Dataset\""
      n105 = in-place {
        in-place-border: [w383] -> w354
        in-place-border: [w381] -> w349
        n106 = in-place-dvr #4(w351) -> (w382:T45, w381:errorcluster)
        n107 = Unbundle By Name(w382) -> ("Single Data Point Path"=w383:path)
        n108 = in-place-dvr #4() -> (w350:refnum<data-value>)  [unwired: 1 in, 1 out]
      }
      n109 = Unbundle By Name(w358) -> ("Dataset Control References.Current Data"=w357:refnum<vi>, "Dataset Control References.Time Point Slide"=w356:refnum<vi>)
      n110 = Variant To Data(error in=w349, type=T18 {"FLI Dataset Type"=enum."HDF5 FLI Dataset", "No Dialog?"=FALSE, "File Path"=path ""} ("output cluster"), Variant=w373) -> (data=w371:T18, error out=w348:errorcluster)
      n111 = Unbundle By Name(w358) -> ("Phasor Plot Ctrl Refnums.Save Phasor Plot"=w362:refnum<vi>, "Dataset Control References.Save Image"=w360:refnum<vi>, "Dataset Control References.Displayed Image"=w353:refnum<vi>)
      n112 = case shown="Error .." w348 {
        selector: w348 -> [w375 _]
        tunnel: w371 -> [w378 _]
        tunnel: [w377 AlliGator_FLI_Dataset_Type."HDF5 FLI Dataset" ("FLI Dataset Type")] -> w370
        tunnel: [w376 TRUE ("No Dialog?")] -> w369
        tunnel: [w375 _] -> w347
        frame No Error {
          n113 = Unbundle By Name(w378) -> ("No Dialog?"=w376:bool, "FLI Dataset Type"=w377:T19)
        }
        frame Error {
          # "#TODO: pass dataset type"
        }
      }
      n114 = property class="Enum (strict)"(reference=w353) -> ("Value"=w352:T75)  [unwired: 1 in, 2 out]
      n115 = property class="Bool (strict)"(reference=w362) -> ("Value"=w361:bool)  [unwired: 1 in, 2 out]
      n116 = property class="Bool (strict)"(reference=w360) -> ("Value"=w359:bool)  [unwired: 1 in, 2 out]
      n117 = property class="Str"(reference=w357, "Visible"=w355) -> ()  [unwired: 1 in, 2 out]
      n118 = property class="Slide (strict)"(reference=w356, "Visible"=w355) -> ()  [unwired: 1 in, 2 out]
      n119 = call "AlliGator Script_Open Single FLI Dataset.vi"("Type of Displayed Image"=w352, "FLI Dataset Type"=w370, "No Dialog? (T)"=w369, "File Path"=w354, "Save Image with Overlay"=w361, "Error In"=w347, "Save Phasor Plot with Overlay"=w359) -> ("Action List out"=w367:T5[], "Error Out"=w365:errorcluster)  [unwired: 7 in]
      n120 = call-poly "AlliGator Add Action(s) to Stack.vi"("Elements Order in Action Stack (Default: 2 BEFORE 1)"=Alligator_Elements_Order_in_Action_Stack."Enqueue 2 BEFORE 1", "Error In"=w365, "Alligator Queue Element 2"=w367, "Alligator Queue Element 1"=w368) -> ("Error Out"=w364:errorcluster, "Alligator Queue Element 1 (+ 2)"=w366:T5[])  [unwired: 6 in]
    }
    frame "Files:Open White Light Image" {
      # "\"Open Single Image\""
      n121 = call "AlliGator Script Open White Light Image.vi"("Image Path"=path "") -> ("Error Out"=w387:errorcluster, "Action List out"=w389:T5[])  [unwired: 9 in]
      n122 = call-poly "AlliGator Add Action(s) to Stack.vi"("Elements Order in Action Stack (Default: 2 BEFORE 1)"=Alligator_Elements_Order_in_Action_Stack."Enqueue 2 BEFORE 1", "Error In"=w387, "Alligator Queue Element 2"=w389, "Alligator Queue Element 1"=w390) -> ("Error Out"=w386:errorcluster, "Alligator Queue Element 1 (+ 2)"=w388:T5[])  [unwired: 6 in]
    }
    frame "Files:Save Mask Image" {
      # "\"Files:Save Mask Image\""
      n123 = call "AlliGator Save Mask Image.vi"("error in (no error)"=w394, "AlliGator IV DVR in"=w397) -> ("error out"=w395:errorcluster, "Message"=w393:string, "AlliGator IV DVR out"=w396:refnum<data-value>)  [unwired: 7 in]
    }
    frame "Files:Select Folder" {
      # "\"Select Folder\""
      n124 = Variant To Data(type=T22 {"Folder Selection Mode"=enum."Select Gate Folder", "Folder Path"=path ""} ("Folder Selection"), Variant=w413) -> (data=w407:T22, error out=w401:errorcluster)  [unwired: 1 in]
      n125 = case shown="Error .." w401 {
        selector: w401 -> [w419 _]
        tunnel: w407 -> [w422 _]
        tunnel: [w421 _] -> w406
        tunnel: [w420 AlliGator_Select_Folder_Mode."Select Folder of HDF5 FLI Datasets" ("Folder Selection Mode")] -> w402
        tunnel: [w419 _] -> w400
        frame No Error {
          n126 = Unbundle By Name(w422) -> ("Folder Path"=w421:path, "Folder Selection Mode"=w420:T23)
        }
        frame Error {
          # "#TODO: pass folder path and type"
        }
      }
      n127 = call "AlliGator Select Folder.vi"("Error In"=w400, "Folder Selection Mode"=w402, "Folder Path"=w406, "AlliGator IV DVR in"=w404) -> ("Error Out"=w403:errorcluster, "cancelled"=w416:bool, "selected path"=w412:path, "AlliGator IV DVR out"=w405:refnum<data-value>, "AlliGator Q Element"=w409:T5)  [unwired: 3 in]
      n128 = case shown="False" w416 {
        tunnel: w418 -> [w432 w436]
        tunnel: [w431 w436] -> w417
        tunnel: w409 -> [w428 _]
        tunnel: w414 -> [w429 _]
        tunnel: w412 -> [w426 _]
        tunnel: w411 -> [w427 _]
        tunnel: w403 -> [w425 w435]
        tunnel: [w424 w434] -> w410
        frame False {
          n129 = call "Add File Path to VI Title.vi"("Error In"=w425, "VI Title"=w427, "File Path"=w426, "VI Refnum"=w429) -> ("Error Out"=w424:errorcluster)  [unwired: 7 in]
          n130 = call-poly "AlliGator Add Action(s) to Stack.vi"("Elements Order in Action Stack (Default: 2 BEFORE 1)"=Alligator_Elements_Order_in_Action_Stack."Enqueue 2 BEFORE 1", "Alligator Atomic Action"=w428, "Alligator Queue Element 1"=w432) -> ("Alligator Queue Element 1 (+ 2)"=w431:T5[])  [unwired: 7 in, 1 out]
        }
        frame True {
          w433 = 43  # Operation cancelled by user
          n131 = call <vilib>:"Clear Errors.vi"("error in (no error)"=w435, "specific error code to clear (0: all)"=w433) -> ("error out"=w434:errorcluster)  [unwired: 4 in, 1 out]
        }
      }
    }
    frame "Files:Set Batch Export Files To Save" {
      # "\"Set Batch Export File To Save\""
      n132 = call-poly "Variant to Data.vi"("Variant"=w444) -> ("Path"=w441:path)  [unwired: 8 in]
      n133 = call "AlliGator Batch Export Status.vi"("Set/Get (F)"=FALSE) -> ("error out"=w438:errorcluster, "Conversion Jobs out"=w442:T76[])  [unwired: 9 in]
      n134 = for {
        tunnel: w442 -> [w452] mode=indexing
        tunnel: w441 -> [w453]
        tunnel: [w449] -> w440 mode=indexing
        n135 = Unbundle By Name(w452) -> ("File Path"=w454:path, "Saved"=w451:bool)
        n136 = Equal?(x=w453, y=w454) -> (x = y?=w450:bool)
        n137 = Or(x=w450, y=w451) -> (x .or. y?=w448:bool)
        n138 = Bundle By Name(cluster=w452, "Saved"=w448) -> (w449:T76)
      }
      n139 = call "AlliGator Batch Export Status.vi"("Set/Get (F)"=TRUE, "error in (no error)"=w438, "Conversion Jobs in"=w440) -> ()  [unwired: 7 in, 2 out]
    }
    frame "Files:Set Dataset Loading & Pre-processing Options" {
      # "\"Set Dataset Loading & Pre-processing Options\""
      n140 = Variant To Data(type=T24 {"Data Information"={"Gates to Skip"={"Start"=0, "End"=0}, "# Gates"=1, "Gate Step"=1, "Gate Duration"=3e-10, "Gate Separation"=4e-11, "Pile-up Correction"=FALSE, "Pixel Well Capacity"=1, "Define Gates to"=enum."Skip", "Gates to Keep"={"First"=0, "Last"=0}, "Laser Period"=0.0, "SYNC Period"=0.0, "Channel Name"=0, "Channel Arithmetic"=enum."None", "Background File Subtraction"=FALSE, "Background Scaling Factor"=1.0, "Background File"=path "", "Background Pile-up Correction"=FALSE, "Background Pixel Well Capacity"=1, "Dataset Scaling Factor"=1.0}, "Source Image Settings"={"Low Count Pixels Rejection Options"={"Background Low Threshold Factor"=0.0, "Fixed Low Background Threshold"=20000.0, "Reject Low Count Pixels"=FALSE, "Low Percentile"=0.0}, "High Count Pixels Rejection Options"={"Background High Threshold Factor"=0.0, "Fixed High Background Threshold"=1.0, "Reject High Count Pixels"=FALSE, "High Percentile"=100.0}, "Peak Threshold"=500.0, "Intensity Threshold"=500.0, "Image Smoothing Options"={"Use Image Smoothing"=FALSE, "Kernel Type"=enum."Bilinear", "Bin"=1, "Algorithm"=enum."Rapid"}, "Image Binning Options"={"Use Image Binning"=FALSE, "X Bin"=1, "Y Bin"=1}}, "Decay Preprocessing Options & Parameters"={"Background Subtraction Parameters"={"Background Definition Range"={"Min Gate"=0.0, "Max Gate"=0.0}, "Baseline Subtraction Method"=enum."Mean", "Background Subtraction?"=FALSE, "Background File"=path "", "Background Constant"=0.0, "Background Scaling Factor"=1.0, "Background Pile-up Correction"=FALSE, "Background Pixel Well Capacity"=1}, "Decay Preprocessing Parameters"={"Background Subtraction"=FALSE, "Straighten Decay"=FALSE, "Reverse Gates"=FALSE, "1-Normalized Decay"=FALSE, "Smoothen Decay"=FALSE, "Smoothing Parameter"=0.0, "Shift Decay"=FALSE, "Decay Shift Parameters"={"Type"=enum."Default", "Shift"=0.0, "Threshold"=0.0, "Rotate"=FALSE}, "Extrapolate Decay"=FALSE, "Additional Points"=0, "Head Fraction"=0.0, "Pixel-Normalize Decay"=FALSE, "Use Periodicity"=FALSE, "Use Cursors"=FALSE, "Tail Fraction"=0.0, "Use Decay Pre-Processing"=TRUE, "Fold Decay"=FALSE, "# Folds"=1, "[0-1]-Normalized Decay"=FALSE}, "Preprocessing Steps Order"=[]}, "Clear Phasor Graph"=FALSE} ("Dataset Loading & Pre-processing Options"), Variant=w461) -> (data=w459:T24, error out=w458:errorcluster)  [unwired: 1 in]
      n141 = call "AlliGator Get-Set Loading & Pre-Processing Options.vi"("Get (F)/Set"=TRUE, "Error In"=w458, "Dataset Loading & Pre-processing Options (in)"=w459) -> ("Error Out"=w456:errorcluster)  [unwired: 7 in, 1 out]
    }
    frame "Files:Set Destination File Path" {
      # "\"Set Destination File Path\""
      n142 = call-poly "Variant to Data.vi"("Variant"=w469) -> ("Path"=w468:path)  [unwired: 8 in]
      n143 = call "Alligator Variables Storage.vi"("Get(F)/Set"=TRUE, "AlliGator Variable"=AlliGator_Variables_List."Destination File Path" ("Alligator Variable"), "Data in"=w468) -> ("Error Out"=w465:errorcluster)  [unwired: 6 in, 2 out]
    }
    frame "Files:Subtract Background File" {
      # "\"Subtract Background File\""
      n144 = call-poly "Variant to Data.vi"("Variant"=w486) -> ("Path"=w482:path)  [unwired: 8 in]
      n145 = call "Show Animated Busy Icon with Message.vi"("Already active? (F)"=w473, "Message"=w475, "Target VI Refnum"=w480) -> ("Error Out"=w479:errorcluster)  [unwired: 8 in]
      n146 = call "AlliGator Get Background File Data v2.vi"("Error In"=w479, "Path"=w482, "AlliGator IV DVR in"=w477) -> ("Error Out"=w488:errorcluster, "Background Gate Images, Max & Sum 2"=w483:T47, "Background Gate Images, Max & Sum 1"=w484:T47, "AlliGator IV DVR out"=w485:refnum<data-value>, "Message"=w472:string)  [unwired: 4 in]
      n147 = case shown="No Error" w488 {
        selector: w488 -> [_ w505]
        tunnel: w485 -> [w496 w504]
        tunnel: w484 -> [w494 _]
        tunnel: w483 -> [w493 _]
        tunnel: w482 -> [w501 _]
        tunnel: [w490 w505] -> w476
        tunnel: [w497 w504] -> w478
        tunnel: [w491 w503] -> w474
        tunnel: w472 -> [w489 w503]
        frame No Error {
          n148 = call "AlliGator Settings Storage.vi"("AlliGator Settings List"=AlliGator_Settings_List."Data Information:Background Scaling Factor") -> ("Error Out"=w495:errorcluster, "Variant Data out"=w499:variant)  [unwired: 9 in]
          n149 = call-poly "Variant to Data.vi"("Variant"=w499) -> ("Value"=w492:dbl)  [unwired: 8 in]
          n150 = call "AlliGator Subtract Background Image(s) v4.vi"("error in (no error)"=w495, "Background Gate Images, Min, Max & Sum 2"=w493, "Background Gate Images, Min, Max & Sum 1"=w494, "AlliGator IV DVR in"=w496) -> ("error out"=w498:errorcluster, "AlliGator IV DVR out"=w497:refnum<data-value>)  [unwired: 6 in]
          n151 = Format Into String(format string="\nSubtracted background file: %s\nScaling Factor: %#g", initial string=w489, error in=w498, w501, w492) -> (resulting string=w491:string, error out=w490:errorcluster)
        }
        frame Error {
        }
      }
      n152 = call "Hide Animated Busy Icon with Message and Abort Button.vi"("Already active? (F)"=w473, "Target VI reference"=w480, "Error In"=w476) -> ("Error Out"=w481:errorcluster)  [unwired: 16 in]
    }
  }
  "error out" <- w5
  "Script out" <- w13
  "AlliGator Q Elements out" <- w12
  "AlliGator IV DVR" <- w7
  n153 = call "Message Style.vi"() -> ("Message Formatting"=w2:T3)
  n154 = call "AlliGator Package Notebook Messages.vi"("Message Formatting"=w2, "Message"=w3, "AlliGator Q Event in"="AlliGator Q Event in") -> ("[Notebook Message]"=→"[Notebook Message]":T2[])  [unwired: 8 in]
